vi "BuildRectangularScan_softturn.vi"(0 "VektorCluster":T3={"StartPunkt [m]"={"x"=-3.058577531863264e-05, "y"=1.835670165073038e-05}, "ZeilenIncrement [m]"={"x"=1.0229073667902263e-07, "y"=-4.894247696936301e-07}, "Zeile [m/s]"={"x"=0.21752211986383552, "y"=0.04546254963512117}, "Zeit/Zeile [s]"=0.000225}, 1 "ParameterCluster":T5={"x Pixel"=250, "Lines"=250, "Bidirektional"=TRUE, "AD-Frequency [Hz]"=4000000.0, "Galvo Cycle [s]"=1e-05, "Smartmovedelay [s]"=0.00119, "max.accel. [m/s^2]"=270000.0}) -> (2 "ScanSteuerung":T4(array[cluster])=[{"Zeitpunkt [s]"=0.0, "Wirkung"=enum."Abs", "Kanal"=enum."SMoveTime", "Wert (/s)"=0.0}, {"Zeitpunkt [s]"=0.0, "Wirkung"=enum."Abs", "Kanal"=enum."GalvoX", "Wert (/s)"=-3.058577531863264e-05}, {"Zeitpunkt [s]"=0.0, "Wirkung"=enum."Abs", "Kanal"=enum."GalvoY", "Wert (/s)"=1.835670165073038e-05}, {"Zeitpunkt [s]"=0.0, "Wirkung"=enum."Abs", "Kanal"=enum."Image1X", "Wert (/s)"=0.0}, {"Zeitpunkt [s]"=0.0, "Wirkung"=enum."Abs", "Kanal"=enum."Image1Y", "Wert (/s)"=0.0}, {"Zeitpunkt [s]"=0.0, "Wirkung"=enum."Abs", "Kanal"=enum."Digital", "Wert (/s)"=7.0}, {"Zeitpunkt [s]"=0.0, "Wirkung"=enum."LoopStart", "Kanal"=enum."Loop", "Wert (/s)"=49.0}, {"Zeitpunkt [s]"=0.0, "Wirkung"=enum."Inc", "Kanal"=enum."GalvoX", "Wert (/s)"=0.21752211986383552}, {"Zeitpunkt [s]"=0.0, "Wirkung"=enum."Inc", "Kanal"=enum."GalvoY", "Wert (/s)"=0.04546254963512117}, {"Zeitpunkt [s]"=0.0, "Wirkung"=enum."IncInc", "Kanal"=enum."GalvoX", "Wert (/s)"=0.0}, {"Zeitpunkt [s]"=0.0, "Wirkung"=enum."IncInc", "Kanal"=enum."GalvoY", "Wert (/s)"=0.0}, {"Zeitpunkt [s]"=0.0, "Wirkung"=enum."Inc", "Kanal"=enum."Image1X", "Wert (/s)"=444444.44444444444}, {"Zeitpunkt [s]"=0.00022275, "Wirkung"=enum."Inc", "Kanal"=enum."Image1X", "Wert (/s)"=0.0}, {"Zeitpunkt [s]"=0.000225, "Wirkung"=enum."Inc", "Kanal"=enum."Image1X", "Wert (/s)"=-2315789.47368421}, {"Zeitpunkt [s]"=0.000225, "Wirkung"=enum."Rel", "Kanal"=enum."Image1Y", "Wert (/s)"=1.0}, {"Zeitpunkt [s]"=0.00023, "Wirkung"=enum."Abs", "Kanal"=enum."Digital", "Wert (/s)"=5.0}, {"Zeitpunkt [s]"=0.00023, "Wirkung"=enum."IncInc", "Kanal"=enum."GalvoX", "Wert (/s)"=-146143.4081327828}, {"Zeitpunkt [s]"=0.00023, "Wirkung"=enum."IncInc", "Kanal"=enum."GalvoY", "Wert (/s)"=-32321.565855881716}, {"Zeitpunkt [s]"=0.00025, "Wirkung"=enum."IncInc", "Kanal"=enum."GalvoX", "Wert (/s)"=146143.4081327828}, {"Zeitpunkt [s]"=0.00025, "Wirkung"=enum."IncInc", "Kanal"=enum."GalvoY", "Wert (/s)"=32321.565855881716}, {"Zeitpunkt [s]"=0.00026775000000000003, "Wirkung"=enum."Inc", "Kanal"=enum."Image1X", "Wert (/s)"=0.0}, {"Zeitpunkt [s]"=0.00027, "Wirkung"=enum."Abs", "Kanal"=enum."Digital", "Wert (/s)"=7.0}, {"Zeitpunkt [s]"=0.00027, "Wirkung"=enum."LoopEnd", "Kanal"=enum."Loop", "Wert (/s)"=0.0}, {"Zeitpunkt [s]"=0.01323, "Wirkung"=enum."Inc", "Kanal"=enum."GalvoX", "Wert (/s)"=0.21752211986383552}, {"Zeitpunkt [s]"=0.01323, "Wirkung"=enum."Inc", "Kanal"=enum."GalvoY", "Wert (/s)"=0.04546254963512117}, {"Zeitpunkt [s]"=0.01323, "Wirkung"=enum."IncInc", "Kanal"=enum."GalvoX", "Wert (/s)"=0.0}, {"Zeitpunkt [s]"=0.01323, "Wirkung"=enum."IncInc", "Kanal"=enum."GalvoY", "Wert (/s)"=0.0}, {"Zeitpunkt [s]"=0.01323, "Wirkung"=enum."Inc", "Kanal"=enum."Image1X", "Wert (/s)"=444444.44444444444}, {"Zeitpunkt [s]"=0.013452750000000001, "Wirkung"=enum."Inc", "Kanal"=enum."Image1X", "Wert (/s)"=0.0}, {"Zeitpunkt [s]"=0.013455, "Wirkung"=enum."Inc", "Kanal"=enum."GalvoX", "Wert (/s)"=0.0}, {"Zeitpunkt [s]"=0.013455, "Wirkung"=enum."Inc", "Kanal"=enum."GalvoY", "Wert (/s)"=0.0}, {"Zeitpunkt [s]"=0.013455, "Wirkung"=enum."Abs", "Kanal"=enum."Digital", "Wert (/s)"=0.0}], 3 "Total time":dbl=0.013455, 4 "Line+Turn [s]":dbl=0.00027 format="%^#_6g")   [LabVIEW 2011]
panel:
  out "Galvo tun cycles":dbl=4.0
  out "turn [s] estimate":dbl=0.0004326610977478994
  in  "Neues Zeitraster 2":dbl=1e-05
  in  "Aktiv 2":T1(array[ring])=[enum."GalvoX", enum."GalvoY"]
  out "Fehler":dbl[](array[numeric])=[8.394600298729658e-06, -8.051345387642523e-06]
  out "last value 2":dbl[](array[numeric])=[2.2281337148683577e-05, 4.3766488554712015e-06]
  out "last value":dbl[](array[numeric])=[3.0675937447413235e-05, -3.6746965321713216e-06]
  out "expected classics bidirectioanl":dbl[][](graph)
  in  "Neues Zeitraster":dbl=1e-05
  out "test Graph":dbl[][](graph)=[[-3.058577531863264e-05, 1.835670165073038e-05], [-2.841055411999428e-05, 1.8811327147081594e-05], [-2.6235332921355925e-05, 1.9265952643432807e-05], [-2.4060111722717568e-05, 1.972057813978402e-05], [-2.188489052407921e-05, 2.0175203636135233e-05], [-1.9709669325440853e-05, 2.0629829132486446e-05], [-1.7534448126802496e-05, 2.108445462883766e-05], [-1.535922692816414e-05, 2.153908012518887e-05], [-1.3184005729525784e-05, 2.1993705621540084e-05], [-1.1008784530887429e-05, 2.2448331117891297e-05], [-8.833563332249073e-06, 2.290295661424251e-05], [-6.658342133610718e-06, 2.3357582110593723e-05], [-4.483120934972363e-06, 2.3812207606944936e-05], [-2.3078997363340074e-06, 2.426683310329615e-05], [-1.3267853769565205e-07, 2.472145859964736e-05], [2.0425426609427033e-06, 2.5176084095998575e-05], [4.217763859581059e-06, 2.5630709592349787e-05], [6.392985058219414e-06, 2.6085335088701e-05], [8.56820625685777e-06, 2.6539960585052213e-05], [1.0743427455496125e-05, 2.6994586081403426e-05], [1.291864865413448e-05, 2.744921157775464e-05], [1.5093869852772835e-05, 2.7903837074105852e-05], [1.726909105141119e-05, 2.8358462570457065e-05], [1.9444312250049546e-05, 2.8813088066808278e-05], [2.1619533448687903e-05, 2.926771356315949e-05], [9.180413834047978e-06, 2.649018247392253e-05], [-1.7873046593870224e-05, 2.04804947990974e-05], [-3.0312166208510148e-05, 1.770296370986044e-05], [-2.813694500987179e-05, 1.8157589206211652e-05], [-2.5961723811233434e-05, 1.8612214702562865e-05], [-2.3786502612595077e-05, 1.9066840198914078e-05], [-2.161128141395672e-05, 1.952146569526529e-05], [-1.9436060215318363e-05, 1.9976091191616504e-05], [-1.7260839016680006e-05, 2.0430716687967716e-05], [-1.508561781804165e-05, 2.088534218431893e-05], [-1.2910396619403295e-05, 2.1339967680670142e-05], [-1.073517542076494e-05, 2.1794593177021355e-05], [-8.559954222126584e-06, 2.2249218673372568e-05], [-6.384733023488229e-06, 2.270384416972378e-05], [-4.209511824849874e-06, 2.3158469666074994e-05], [-2.0342906262115183e-06, 2.3613095162426207e-05], [1.40930572426837e-07, 2.406772065877742e-05], [2.3161517710651923e-06, 2.4522346155128633e-05], [4.491372969703548e-06, 2.4976971651479846e-05], [6.666594168341903e-06, 2.543159714783106e-05], [8.841815366980258e-06, 2.588622264418227e-05], [1.1017036565618614e-05, 2.6340848140533484e-05], [1.3192257764256969e-05, 2.6795473636884697e-05], [1.5367478962895323e-05, 2.725009913323591e-05], [1.754270016153368e-05, 2.7704724629587123e-05], [1.9717921360172037e-05, 2.8159350125938336e-05], [2.1893142558810394e-05, 2.861397562228955e-05], [9.454022944170469e-06, 2.5836444533052588e-05], [-1.7599437483747734e-05, 1.9826756858227454e-05], [-3.0038557098387657e-05, 1.7049225768990494e-05], [-2.78633358997493e-05, 1.7503851265341707e-05], [-2.5688114701110943e-05, 1.795847676169292e-05], [-2.3512893502472586e-05, 1.8413102258044132e-05], [-2.133767230383423e-05, 1.8867727754395345e-05], [-1.9162451105195872e-05, 1.9322353250746558e-05], [-1.6987229906557515e-05, 1.977697874709777e-05], [-1.481200870791916e-05, 2.0231604243448984e-05], [-1.2636787509280804e-05, 2.0686229739800197e-05], [-1.0461566310642449e-05, 2.114085523615141e-05], [-8.286345112004094e-06, 2.1595480732502623e-05], [-6.111123913365738e-06, 2.2050106228853836e-05], [-3.935902714727383e-06, 2.250473172520505e-05], [-1.7606815160890276e-06, 2.295935722155626e-05], [4.145396825493277e-07, 2.3413982717907474e-05], [2.589760881187683e-06, 2.3868608214258687e-05], [4.764982079826038e-06, 2.43232337106099e-05], [6.940203278464394e-06, 2.4777859206961113e-05], [9.115424477102749e-06, 2.5232484703312326e-05], [1.1290645675741104e-05, 2.568711019966354e-05], [1.346586687437946e-05, 2.6141735696014752e-05], [1.5641088073017813e-05, 2.6596361192365965e-05], [1.781630927165617e-05, 2.7050986688717178e-05], [1.9991530470294527e-05, 2.750561218506839e-05], [2.2166751668932885e-05, 2.7960237681419603e-05], [9.72763205429296e-06, 2.5182706592182643e-05], [-1.7325828373625243e-05, 1.917301891735751e-05], [-2.9764947988265166e-05, 1.639548782812055e-05], [-2.758972678962681e-05, 1.685011332447176e-05], [-2.5414505590988452e-05, 1.7304738820822974e-05], [-2.3239284392350095e-05, 1.7759364317174187e-05], [-2.106406319371174e-05, 1.82139898135254e-05], [-1.888884199507338e-05, 1.8668615309876613e-05], [-1.6713620796435024e-05, 1.9123240806227826e-05], [-1.4538399597796669e-05, 1.957786630257904e-05], [-1.2363178399158314e-05, 2.003249179893025e-05], [-1.0187957200519958e-05, 2.0487117295281464e-05], [-8.012736001881603e-06, 2.0941742791632677e-05], [-5.8375148032432476e-06, 2.139636828798389e-05], [-3.6622936046048922e-06, 2.1850993784335103e-05], [-1.4870724059665369e-06, 2.2305619280686316e-05], [6.881487926718185e-07, 2.276024477703753e-05], [2.863369991310174e-06, 2.3214870273388742e-05], [5.038591189948529e-06, 2.3669495769739955e-05], [7.2138123885868845e-06, 2.4124121266091168e-05], [9.38903358722524e-06, 2.457874676244238e-05], [1.1564254785863595e-05, 2.5033372258793593e-05], [1.373947598450195e-05, 2.5487997755144806e-05], [1.5914697183140304e-05, 2.594262325149602e-05], [1.808991838177866e-05, 2.6397248747847232e-05], [2.0265139580417018e-05, 2.6851874244198445e-05], [2.2440360779055375e-05, 2.7306499740549658e-05], [1.000124116441545e-05, 2.4528968651312697e-05], [-1.7052219263502752e-05, 1.8519280976487563e-05], [-2.9491338878142676e-05, 1.5741749887250603e-05], [-2.731611767950432e-05, 1.6196375383601816e-05], [-2.514089648086596e-05, 1.665100087995303e-05], [-2.2965675282227605e-05, 1.710562637630424e-05], [-2.0790454083589248e-05, 1.7560251872655455e-05], [-1.861523288495089e-05, 1.8014877369006667e-05], [-1.6440011686312534e-05, 1.846950286535788e-05], [-1.4264790487674178e-05, 1.8924128361709093e-05], [-1.2089569289035823e-05, 1.9378753858060306e-05], [-9.914348090397468e-06, 1.983337935441152e-05], [-7.739126891759112e-06, 2.0288004850762732e-05], [-5.563905693120757e-06, 2.0742630347113945e-05], [-3.3886844944824015e-06, 2.1197255843465158e-05], [-1.2134632958440462e-06, 2.165188133981637e-05], [9.617579027943092e-07, 2.2106506836167584e-05], [3.1369791014326645e-06, 2.2561132332518797e-05], [5.31220030007102e-06, 2.301575782887001e-05], [7.487421498709375e-06, 2.3470383325221222e-05], [9.66264269734773e-06, 2.3925008821572435e-05], [1.1837863895986086e-05, 2.4379634317923648e-05], [1.4013085094624441e-05, 2.483425981427486e-05], [1.6188306293262795e-05, 2.5288885310626074e-05], [1.8363527491901152e-05, 2.5743510806977287e-05], [2.053874869053951e-05, 2.61981363033285e-05], [2.2713969889177866e-05, 2.6652761799679713e-05], [1.027485027453794e-05, 2.3875230710442752e-05], [-1.677861015338026e-05, 1.7865543035617618e-05], [-2.9217729768020185e-05, 1.5088011946380658e-05], [-2.7042508569381828e-05, 1.554263744273187e-05], [-2.486728737074347e-05, 1.5997262939083083e-05], [-2.2692066172105114e-05, 1.6451888435434296e-05], [-2.0516844973466757e-05, 1.690651393178551e-05], [-1.83416237748284e-05, 1.7361139428136722e-05], [-1.6166402576190043e-05, 1.7815764924487935e-05], [-1.3991181377551687e-05, 1.8270390420839148e-05], [-1.1815960178913332e-05, 1.872501591719036e-05], [-9.640738980274977e-06, 1.9179641413541574e-05], [-7.4655177816366214e-06, 1.9634266909892787e-05], [-5.290296582998266e-06, 2.0088892406244e-05], [-3.1150753843599108e-06, 2.0543517902595212e-05], [-9.398541857215554e-07, 2.0998143398946425e-05], [1.2353670129168e-06, 2.1452768895297638e-05], [3.4105882115551553e-06, 2.190739439164885e-05], [5.585809410193511e-06, 2.2362019888000064e-05], [7.761030608831866e-06, 2.2816645384351277e-05], [9.936251807470221e-06, 2.327127088070249e-05], [1.2111473006108577e-05, 2.3725896377053703e-05], [1.4286694204746932e-05, 2.4180521873404916e-05], [1.6461915403385286e-05, 2.463514736975613e-05], [1.8637136602023643e-05, 2.508977286610734e-05], [2.0812357800662e-05, 2.5544398362458554e-05], [2.2987578999300357e-05, 2.5999023858809767e-05], [1.0548459384660432e-05, 2.3221492769572807e-05], [-1.650500104325777e-05, 1.7211805094747673e-05], [-2.8944120657897694e-05, 1.4434274005510712e-05], [-2.6768899459259337e-05, 1.4888899501861923e-05], [-2.459367826062098e-05, 1.5343524998213135e-05], [-2.2418457061982623e-05, 1.5798150494564348e-05], [-2.0243235863344266e-05, 1.625277599091556e-05], [-1.806801466470591e-05, 1.6707401487266773e-05], [-1.5892793466067552e-05, 1.7162026983617986e-05], [-1.3717572267429197e-05, 1.76166524799692e-05], [-1.1542351068790841e-05, 1.8071277976320412e-05], [-9.367129870152486e-06, 1.8525903472671625e-05], [-7.191908671514131e-06, 1.8980528969022838e-05], [-5.016687472875775e-06, 1.943515446537405e-05], [-2.84146627423742e-06, 1.9889779961725264e-05], [-6.662450755990647e-07, 2.0344405458076477e-05], [1.5089761230392907e-06, 2.079903095442769e-05], [3.684197321677646e-06, 2.1253656450778902e-05], [5.859418520316001e-06, 2.1708281947130115e-05], [8.034639718954357e-06, 2.2162907443481328e-05], [1.0209860917592712e-05, 2.261753293983254e-05], [1.2385082116231067e-05, 2.3072158436183754e-05], [1.4560303314869423e-05, 2.3526783932534967e-05], [1.6735524513507776e-05, 2.398140942888618e-05], [1.8910745712146133e-05, 2.4436034925237393e-05], [2.108596691078449e-05, 2.4890660421588606e-05], [2.3261188109422847e-05, 2.534528591793982e-05], [1.0822068494782922e-05, 2.2567754828702858e-05], [-1.623139193313528e-05, 1.6558067153877727e-05], [-2.8670511547775204e-05, 1.3780536064640767e-05], [-2.6495290349136847e-05, 1.4235161560991978e-05], [-2.432006915049849e-05, 1.468978705734319e-05], [-2.2144847951860132e-05, 1.51444125536944e-05], [-1.9969626753221775e-05, 1.559903805004561e-05], [-1.779440555458342e-05, 1.6053663546396825e-05], [-1.561918435594506e-05, 1.6508289042748037e-05], [-1.3443963157306706e-05, 1.696291453909925e-05], [-1.126874195866835e-05, 1.7417540035450463e-05], [-9.093520760029995e-06, 1.7872165531801676e-05], [-6.91829956139164e-06, 1.832679102815289e-05], [-4.743078362753285e-06, 1.8781416524504102e-05], [-2.5678571641149293e-06, 1.9236042020855315e-05], [-3.9263596547657396e-07, 1.9690667517206528e-05], [1.7825852331617814e-06, 2.014529301355774e-05], [3.957806431800137e-06, 2.0599918509908954e-05], [6.133027630438492e-06, 2.1054544006260167e-05], [8.308248829076847e-06, 2.150916950261138e-05], [1.0483470027715203e-05, 2.1963794998962592e-05], [1.2658691226353558e-05, 2.2418420495313805e-05], [1.4833912424991913e-05, 2.2873045991665018e-05], [1.7009133623630267e-05, 2.332767148801623e-05], [1.9184354822268624e-05, 2.3782296984367444e-05], [2.135957602090698e-05, 2.4236922480718657e-05], [2.3534797219545338e-05, 2.469154797706987e-05], [1.1095677604905413e-05, 2.191401688783291e-05], [-1.595778282301279e-05, 1.5904329213007775e-05], [-2.8396902437652713e-05, 1.3126798123770815e-05], [-2.6221681239014356e-05, 1.3581423620122026e-05], [-2.4046460040376e-05, 1.4036049116473237e-05], [-2.1871238841737642e-05, 1.4490674612824448e-05], [-1.9696017643099285e-05, 1.494530010917566e-05], [-1.7520796444460928e-05, 1.5399925605526872e-05], [-1.534557524582257e-05, 1.5854551101878085e-05], [-1.3170354047184215e-05, 1.6309176598229298e-05], [-1.099513284854586e-05, 1.676380209458051e-05], [-8.819911649907505e-06, 1.7218427590931724e-05], [-6.644690451269149e-06, 1.7673053087282937e-05], [-4.469469252630794e-06, 1.812767858363415e-05], [-2.2942480539924386e-06, 1.8582304079985363e-05], [-1.1902685535408323e-07, 1.9036929576336576e-05], [2.056194343284272e-06, 1.949155507268779e-05], [4.2314155419226275e-06, 1.9946180569039e-05], [6.406636740560983e-06, 2.0400806065390214e-05], [8.581857939199338e-06, 2.0855431561741427e-05], [1.0757079137837693e-05, 2.131005705809264e-05], [1.2932300336476049e-05, 2.1764682554443853e-05], [1.5107521535114404e-05, 2.2219308050795066e-05], [1.7282742733752758e-05, 2.267393354714628e-05], [1.9457963932391115e-05, 2.3128559043497492e-05], [2.1633185131029472e-05, 2.3583184539848705e-05], [2.380840632966783e-05, 2.4037810036199918e-05], [1.1369286715027904e-05, 2.1260278946962957e-05], [-1.56841737128903e-05, 1.5250591272137825e-05], [-2.8123293327530222e-05, 1.2473060182900864e-05], [-2.5948072128891865e-05, 1.2927685679252075e-05], [-2.3772850930253508e-05, 1.3382311175603287e-05], [-2.159762973161515e-05, 1.3836936671954498e-05], [-1.9422408532976794e-05, 1.4291562168305709e-05], [-1.7247187334338437e-05, 1.474618766465692e-05], [-1.5071966135700082e-05, 1.5200813161008132e-05], [-1.2896744937061726e-05, 1.5655438657359343e-05], [-1.0721523738423371e-05, 1.6110064153710556e-05], [-8.546302539785016e-06, 1.656468965006177e-05], [-6.37108134114666e-06, 1.701931514641298e-05], [-4.195860142508305e-06, 1.7473940642764194e-05], [-2.0206389438699495e-06, 1.7928566139115407e-05], [1.545822547684058e-07, 1.838319163546662e-05], [2.329803453406761e-06, 1.8837817131817833e-05], [4.5050246520451165e-06, 1.9292442628169046e-05], [6.680245850683472e-06, 1.974706812452026e-05], [8.855467049321827e-06, 2.0201693620871472e-05], [1.1030688247960183e-05, 2.0656319117222685e-05], [1.3205909446598538e-05, 2.1110944613573898e-05], [1.538113064523689e-05, 2.156557010992511e-05], [1.755635184387525e-05, 2.2020195606276323e-05], [1.9731573042513606e-05, 2.2474821102627536e-05], [2.1906794241151963e-05, 2.292944659897875e-05], [2.408201543979032e-05, 2.3384072095329962e-05], [1.1642895825150394e-05, 2.0606541006093e-05], [-1.5410564602767808e-05, 1.459685333126787e-05], [-2.784968421740773e-05, 1.1819322242030909e-05], [-2.5674463018769374e-05, 1.227394773838212e-05], [-2.3499241820131017e-05, 1.2728573234733331e-05], [-2.132402062149266e-05, 1.3183198731084542e-05], [-1.9148799422854303e-05, 1.3637824227435754e-05], [-1.6973578224215946e-05, 1.4092449723786965e-05], [-1.479835702557759e-05, 1.4547075220138176e-05], [-1.2623135826939235e-05, 1.5001700716489387e-05], [-1.044791462830088e-05, 1.54563262128406e-05], [-8.272693429662525e-06, 1.5910951709191813e-05], [-6.0974722310241695e-06, 1.6365577205543026e-05], [-3.922251032385814e-06, 1.682020270189424e-05], [-1.7470298337474588e-06, 1.7274828198245452e-05], [4.2819136489089654e-07, 1.7729453694596665e-05], [2.603412563529252e-06, 1.8184079190947878e-05], [4.778633762167607e-06, 1.863870468729909e-05], [6.9538549608059626e-06, 1.9093330183650303e-05], [9.129076159444318e-06, 1.9547955680001516e-05], [1.1304297358082673e-05, 2.000258117635273e-05], [1.3479518556721029e-05, 2.0457206672703942e-05], [1.5654739755359382e-05, 2.0911832169055155e-05], [1.782996095399774e-05, 2.1366457665406368e-05], [2.0005182152636096e-05, 2.182108316175758e-05], [2.2180403351274453e-05, 2.2275708658108794e-05], [2.435562454991281e-05, 2.2730334154460007e-05], [1.1916504935272885e-05, 1.9952803065223046e-05], [-1.5136955492645319e-05, 1.3943115390397914e-05], [-2.757607510728524e-05, 1.1165584301160953e-05], [-2.5400853908646884e-05, 1.1620209797512164e-05], [-2.3225632710008527e-05, 1.2074835293863376e-05], [-2.105041151137017e-05, 1.2529460790214587e-05], [-1.8875190312731812e-05, 1.2984086286565798e-05], [-1.6699969114093455e-05, 1.343871178291701e-05], [-1.45247479154551e-05, 1.389333727926822e-05], [-1.2349526716816745e-05, 1.4347962775619432e-05], [-1.017430551817839e-05, 1.4802588271970643e-05], [-7.999084319540034e-06, 1.5257213768321854e-05], [-5.823863120901679e-06, 1.5711839264673067e-05], [-3.6486419222633234e-06, 1.616646476102428e-05], [-1.473420723624968e-06, 1.6621090257375493e-05], [7.018004750133873e-07, 1.7075715753726706e-05], [2.8770216736517426e-06, 1.753034125007792e-05], [5.052242872290098e-06, 1.798496674642913e-05], [7.227464070928453e-06, 1.8439592242780344e-05], [9.402685269566809e-06, 1.8894217739131557e-05], [1.1577906468205164e-05, 1.934884323548277e-05], [1.375312766684352e-05, 1.9803468731833983e-05], [1.5928348865481873e-05, 2.0258094228185196e-05], [1.810357006412023e-05, 2.071271972453641e-05], [2.0278791262758587e-05, 2.1167345220887622e-05], [2.2454012461396944e-05, 2.1621970717238835e-05], [2.46292336600353e-05, 2.2076596213590048e-05], [1.2190114045395376e-05, 1.9299065124353087e-05], [-1.4863346382522828e-05, 1.3289377449527955e-05], [-2.730246599716275e-05, 1.0511846360290994e-05], [-2.5127244798524393e-05, 1.0966471856642205e-05], [-2.2952023599886036e-05, 1.1421097352993417e-05], [-2.077680240124768e-05, 1.1875722849344628e-05], [-1.8601581202609322e-05, 1.2330348345695839e-05], [-1.6426360003970965e-05, 1.278497384204705e-05], [-1.425113880533261e-05, 1.3239599338398262e-05], [-1.2075917606694254e-05, 1.3694224834749473e-05], [-9.900696408055899e-06, 1.4148850331100684e-05], [-7.725475209417543e-06, 1.4603475827451895e-05], [-5.550254010779188e-06, 1.5058101323803106e-05], [-3.3750328121408327e-06, 1.5512726820154318e-05], [-1.1998116135024773e-06, 1.596735231650553e-05], [9.75409585135878e-07, 1.6421977812856743e-05], [3.1506307837742333e-06, 1.6876603309207956e-05], [5.325851982412589e-06, 1.733122880555917e-05], [7.501073181050944e-06, 1.7785854301910382e-05], [9.6762943796893e-06, 1.8240479798261595e-05], [1.1851515578327655e-05, 1.8695105294612808e-05], [1.402673677696601e-05, 1.914973079096402e-05], [1.6201957975604364e-05, 1.9604356287315234e-05], [1.837717917424272e-05, 2.0058981783666447e-05], [2.0552400372881078e-05, 2.051360728001766e-05], [2.2727621571519435e-05, 2.0968232776368872e-05], [2.4902842770157792e-05, 2.1422858272720085e-05], [1.2463723155517867e-05, 1.8645327183483125e-05], [-1.4589737272400337e-05, 1.2635639508657992e-05], [-2.702885688704026e-05, 9.858108419421032e-06], [-2.4853635688401902e-05, 1.0312733915772243e-05], [-2.2678414489763545e-05, 1.0767359412123454e-05], [-2.0503193291125188e-05, 1.1221984908474666e-05], [-1.832797209248683e-05, 1.1676610404825877e-05], [-1.6152750893848474e-05, 1.2131235901177088e-05], [-1.3977529695210119e-05, 1.25858613975283e-05], [-1.1802308496571763e-05, 1.304048689387951e-05], [-9.627087297933408e-06, 1.3495112390230722e-05], [-7.451866099295053e-06, 1.3949737886581933e-05], [-5.276644900656697e-06, 1.4404363382933144e-05], [-3.101423702018342e-06, 1.4858988879284355e-05], [-9.262025033799866e-07, 1.5313614375635568e-05], [1.2490186952583687e-06, 1.576823987198678e-05], [3.424239893896724e-06, 1.6222865368337994e-05], [5.599461092535079e-06, 1.6677490864689207e-05], [7.774682291173435e-06, 1.713211636104042e-05], [9.94990348981179e-06, 1.7586741857391633e-05], [1.2125124688450145e-05, 1.8041367353742846e-05], [1.43003458870885e-05, 1.849599285009406e-05], [1.6475567085726854e-05, 1.895061834644527e-05], [1.865078828436521e-05, 1.9405243842796484e-05], [2.082600948300357e-05, 1.9859869339147697e-05], [2.3001230681641926e-05, 2.031449483549891e-05], [2.5176451880280283e-05, 2.0769120331850123e-05], [1.2737332265640357e-05, 1.7991589242613162e-05], [-1.4316128162277847e-05, 1.198190156778803e-05], [-2.675524777691777e-05, 9.20437047855107e-06], [-2.458002657827941e-05, 9.658995974902281e-06], [-2.2404805379641054e-05, 1.0113621471253492e-05], [-2.0229584181002697e-05, 1.0568246967604703e-05], [-1.805436298236434e-05, 1.1022872463955914e-05], [-1.5879141783725983e-05, 1.1477497960307126e-05], [-1.3703920585087628e-05, 1.1932123456658337e-05], [-1.1528699386449273e-05, 1.2386748953009548e-05], [-9.353478187810917e-06, 1.284137444936076e-05], [-7.178256989172562e-06, 1.329599994571197e-05], [-5.0030357905342065e-06, 1.3750625442063182e-05], [-2.827814591895851e-06, 1.4205250938414393e-05], [-6.525933932574959e-07, 1.4659876434765604e-05], [1.5226278053808595e-06, 1.5114501931116815e-05], [3.697849004019215e-06, 1.5569127427468028e-05], [5.87307020265757e-06, 1.602375292381924e-05], [8.048291401295925e-06, 1.6478378420170454e-05], [1.022351259993428e-05, 1.6933003916521667e-05], [1.2398733798572636e-05, 1.738762941287288e-05], [1.4573954997210992e-05, 1.7842254909224093e-05], [1.6749176195849345e-05, 1.8296880405575306e-05], [1.8924397394487702e-05, 1.875150590192652e-05], [2.109961859312606e-05, 1.920613139827773e-05], [2.3274839791764416e-05, 1.9660756894628944e-05], [2.5450060990402773e-05, 2.0115382390980157e-05], [1.3010941375762848e-05, 1.7337851301743197e-05], [-1.4042519052155356e-05, 1.1328163626918064e-05], [-2.6481638666795278e-05, 8.550632537681104e-06], [-2.430641746815692e-05, 9.005258034032315e-06], [-2.2131196269518564e-05, 9.459883530383526e-06], [-1.9955975070880207e-05, 9.914509026734738e-06], [-1.778075387224185e-05, 1.0369134523085949e-05], [-1.5605532673603493e-05, 1.082376001943716e-05], [-1.3430311474965137e-05, 1.1278385515788371e-05], [-1.1255090276326782e-05, 1.1733011012139582e-05], [-9.079869077688426e-06, 1.2187636508490794e-05], [-6.904647879050071e-06, 1.2642262004842005e-05], [-4.729426680411716e-06, 1.3096887501193216e-05], [-2.5542054817733605e-06, 1.3551512997544427e-05], [-3.7898428313500514e-07, 1.4006138493895638e-05], [1.7962369155033502e-06, 1.446076399024685e-05], [3.9714581141417055e-06, 1.4915389486598061e-05], [6.146679312780061e-06, 1.5370014982949272e-05], [8.321900511418416e-06, 1.5824640479300485e-05], [1.0497121710056772e-05, 1.6279265975651698e-05], [1.2672342908695127e-05, 1.673389147200291e-05], [1.4847564107333482e-05, 1.7188516968354124e-05], [1.7022785305971836e-05, 1.7643142464705337e-05], [1.9198006504610193e-05, 1.809776796105655e-05], [2.137322770324855e-05, 1.8552393457407762e-05], [2.3548448901886907e-05, 1.9007018953758975e-05], [2.5723670100525264e-05, 1.9461644450110188e-05], [1.3284550485885339e-05, 1.6684113360873228e-05], [-1.3768909942032865e-05, 1.0674425686048095e-05], [-2.6208029556672787e-05, 7.896894596811135e-06], [-2.403280835803443e-05, 8.351520093162346e-06], [-2.1857587159396073e-05, 8.806145589513557e-06], [-1.9682365960757716e-05, 9.260771085864769e-06], [-1.750714476211936e-05, 9.71539658221598e-06], [-1.5331923563481002e-05, 1.0170022078567191e-05], [-1.3156702364842646e-05, 1.0624647574918402e-05], [-1.0981481166204291e-05, 1.1079273071269613e-05], [-8.806259967565936e-06, 1.1533898567620825e-05], [-6.63103876892758e-06, 1.1988524063972036e-05], [-4.455817570289225e-06, 1.2443149560323247e-05], [-2.2805963716508697e-06, 1.2897775056674458e-05], [-1.053751730125144e-07, 1.335240055302567e-05], [2.069846025625841e-06, 1.380702604937688e-05], [4.245067224264196e-06, 1.4261651545728092e-05], [6.420288422902552e-06, 1.4716277042079303e-05], [8.595509621540907e-06, 1.5170902538430514e-05], [1.0770730820179262e-05, 1.5625528034781725e-05], [1.2945952018817618e-05, 1.608015353113294e-05], [1.5121173217455973e-05, 1.653477902748415e-05], [1.7296394416094327e-05, 1.6989404523835364e-05], [1.9471615614732684e-05, 1.7444030020186577e-05], [2.164683681337104e-05, 1.789865551653779e-05], [2.3822058012009398e-05, 1.8353281012889003e-05], [2.5997279210647755e-05, 1.8807906509240216e-05], [1.355815959600783e-05, 1.6030375420003255e-05], [-1.3495300831910374e-05, 1.0020687745178123e-05], [-2.5934420446550296e-05, 7.243156655941162e-06], [-2.375919924791194e-05, 7.697782152292374e-06], [-2.1583978049273582e-05, 8.152407648643585e-06], [-1.9408756850635225e-05, 8.607033144994796e-06], [-1.7233535651996868e-05, 9.061658641346007e-06], [-1.5058314453358513e-05, 9.516284137697218e-06], [-1.2883093254720157e-05, 9.97090963404843e-06], [-1.0707872056081802e-05, 1.0425535130399641e-05], [-8.532650857443447e-06, 1.0880160626750852e-05], [-6.357429658805091e-06, 1.1334786123102063e-05], [-4.182208460166736e-06, 1.1789411619453274e-05], [-2.0069872615283807e-06, 1.2244037115804486e-05], [1.6823393710997463e-07, 1.2698662612155697e-05], [2.34345513574833e-06, 1.3153288108506908e-05], [4.518676334386685e-06, 1.360791360485812e-05], [6.693897533025041e-06, 1.406253910120933e-05], [8.869118731663396e-06, 1.4517164597560542e-05], [1.1044339930301751e-05, 1.4971790093911753e-05], [1.3219561128940107e-05, 1.5426415590262966e-05], [1.539478232757846e-05, 1.588104108661418e-05], [1.7570003526216817e-05, 1.633566658296539e-05], [1.9745224724855174e-05, 1.6790292079316605e-05], [2.192044592349353e-05, 1.7244917575667817e-05], [2.409566712213189e-05, 1.769954307201903e-05], [2.6270888320770245e-05, 1.8154168568370243e-05], [1.383176870613032e-05, 1.5376637479133283e-05], [-1.3221691721787884e-05, 9.36694980430815e-06], [-2.5660811336427805e-05, 6.58941871507119e-06], [-2.348559013778945e-05, 7.044044211422402e-06], [-2.131036893915109e-05, 7.498669707773614e-06], [-1.9135147740512734e-05, 7.953295204124825e-06], [-1.6959926541874377e-05, 8.407920700476036e-06], [-1.4784705343236022e-05, 8.862546196827248e-06], [-1.2609484144597667e-05, 9.317171693178459e-06], [-1.0434262945959311e-05, 9.77179718952967e-06], [-8.259041747320956e-06, 1.0226422685880881e-05], [-6.083820548682601e-06, 1.0681048182232093e-05], [-3.908599350044245e-06, 1.1135673678583304e-05], [-1.73337815140589e-06, 1.1590299174934515e-05], [4.4184304723246537e-07, 1.2044924671285726e-05], [2.6170642458708207e-06, 1.2499550167636937e-05], [4.792285444509176e-06, 1.2954175663988149e-05], [6.967506643147531e-06, 1.340880116033936e-05], [9.142727841785887e-06, 1.3863426656690571e-05], [1.1317949040424242e-05, 1.4318052153041782e-05], [1.3493170239062597e-05, 1.4772677649392993e-05], [1.566839143770095e-05, 1.5227303145744205e-05], [1.7843612636339308e-05, 1.5681928642095416e-05], [2.0018833834977665e-05, 1.613655413844663e-05], [2.2194055033616022e-05, 1.659117963479784e-05], [2.436927623225438e-05, 1.7045805131149055e-05], [2.6544497430892736e-05, 1.7500430627500267e-05], [1.4105377816252811e-05, 1.4722899538263307e-05], [-1.2948082611665393e-05, 8.713211863438175e-06], [-2.5387202226305315e-05, 5.935680774201214e-06], [-2.3211981027666958e-05, 6.390306270552426e-06], [-2.10367598290286e-05, 6.844931766903638e-06], [-1.8861538630390244e-05, 7.29955726325485e-06], [-1.6686317431751887e-05, 7.754182759606062e-06], [-1.4511096233113531e-05, 8.208808255957273e-06], [-1.2335875034475176e-05, 8.663433752308485e-06], [-1.016065383583682e-05, 9.118059248659696e-06], [-7.985432637198465e-06, 9.572684745010907e-06], [-5.81021143856011e-06, 1.0027310241362118e-05], [-3.6349902399217546e-06, 1.048193573771333e-05], [-1.4597690412833992e-06, 1.093656123406454e-05], [7.154521573549561e-07, 1.1391186730415752e-05], [2.8906733559933114e-06, 1.1845812226766963e-05], [5.065894554631667e-06, 1.2300437723118174e-05], [7.241115753270022e-06, 1.2755063219469386e-05], [9.416336951908377e-06, 1.3209688715820597e-05], [1.1591558150546733e-05, 1.3664314212171808e-05], [1.3766779349185088e-05, 1.411893970852302e-05], [1.5942000547823442e-05, 1.457356520487423e-05], [1.81172217464618e-05, 1.5028190701225442e-05], [2.0292442945100156e-05, 1.5482816197576653e-05], [2.2467664143738513e-05, 1.5937441693927866e-05], [2.464288534237687e-05, 1.639206719027908e-05], [2.6818106541015227e-05, 1.684669268663029e-05], [1.4378986926375302e-05, 1.4069161597393331e-05], [-1.2674473501542902e-05, 8.059473922568199e-06], [-2.5113593116182824e-05, 5.281942833331238e-06], [-2.2938371917544467e-05, 5.73656832968245e-06], [-2.076315071890611e-05, 6.191193826033662e-06], [-1.8587929520267753e-05, 6.645819322384874e-06], [-1.6412708321629396e-05, 7.1004448187360864e-06], [-1.423748712299104e-05, 7.5550703150872985e-06], [-1.2062265924352685e-05, 8.00969581143851e-06], [-9.88704472571433e-06, 8.464321307789722e-06], [-7.711823527075975e-06, 8.918946804140933e-06], [-5.536602328437619e-06, 9.373572300492144e-06], [-3.361381129799264e-06, 9.828197796843355e-06], [-1.1861599311609085e-06, 1.0282823293194567e-05], [9.890612674774468e-07, 1.0737448789545778e-05], [3.164282466115802e-06, 1.1192074285896989e-05], [5.3395036647541575e-06, 1.16466997822482e-05], [7.514724863392513e-06, 1.2101325278599411e-05], [9.689946062030868e-06, 1.2555950774950623e-05], [1.1865167260669224e-05, 1.3010576271301834e-05], [1.4040388459307579e-05, 1.3465201767653045e-05], [1.6215609657945933e-05, 1.3919827264004256e-05], [1.839083085658429e-05, 1.4374452760355467e-05], [2.0566052055222647e-05, 1.4829078256706679e-05], [2.2741273253861004e-05, 1.528370375305789e-05], [2.491649445249936e-05, 1.5738329249409103e-05], [2.7091715651137718e-05, 1.6192954745760316e-05], [1.4652596036497793e-05, 1.3415423656523355e-05], [-1.2400864391420411e-05, 7.405735981698223e-06], [-2.4839984006060333e-05, 4.628204892461262e-06], [-2.2664762807421976e-05, 5.082830388812474e-06], [-2.048954160878362e-05, 5.5374558851636865e-06], [-1.8314320410145262e-05, 5.9920813815148985e-06], [-1.6139099211506905e-05, 6.4467068778661106e-06], [-1.396387801286855e-05, 6.901332374217323e-06], [-1.1788656814230194e-05, 7.355957870568535e-06], [-9.613435615591839e-06, 7.810583366919746e-06], [-7.438214416953484e-06, 8.265208863270957e-06], [-5.2629932183151285e-06, 8.719834359622168e-06], [-3.087772019676773e-06, 9.17445985597338e-06], [-9.125508210384178e-07, 9.62908535232459e-06], [1.2626703775999376e-06, 1.0083710848675802e-05], [3.437891576238293e-06, 1.0538336345027013e-05], [5.613112774876648e-06, 1.0992961841378224e-05], [7.788333973515004e-06, 1.1447587337729436e-05], [9.963555172153359e-06, 1.1902212834080647e-05], [1.2138776370791714e-05, 1.2356838330431858e-05], [1.431399756943007e-05, 1.281146382678307e-05], [1.6489218768068423e-05, 1.326608932313428e-05], [1.866443996670678e-05, 1.3720714819485492e-05], [2.0839661165345137e-05, 1.4175340315836703e-05], [2.3014882363983494e-05, 1.4629965812187914e-05], [2.519010356262185e-05, 1.5084591308539125e-05], [2.736532476126021e-05, 1.5539216804890336e-05], [1.4926205146620283e-05, 1.2761685715653376e-05], [-1.212725528129792e-05, 6.751998040828244e-06], [-2.4566374895937843e-05, 3.974466951591283e-06], [-2.2391153697299486e-05, 4.429092447942495e-06], [-2.021593249866113e-05, 4.883717944293707e-06], [-1.804071130002277e-05, 5.338343440644919e-06], [-1.5865490101384414e-05, 5.792968936996131e-06], [-1.3690268902746059e-05, 6.247594433347343e-06], [-1.1515047704107704e-05, 6.7022199296985554e-06], [-9.339826505469348e-06, 7.1568454260497675e-06], [-7.164605306830993e-06, 7.6114709224009795e-06], [-4.989384108192638e-06, 8.06609641875219e-06], [-2.8141629095542824e-06, 8.520721915103402e-06], [-6.38941710915927e-07, 8.975347411454613e-06], [1.5362794877224283e-06, 9.429972907805824e-06], [3.7115006863607836e-06, 9.884598404157036e-06], [5.886721884999139e-06, 1.0339223900508247e-05], [8.061943083637494e-06, 1.0793849396859458e-05], [1.023716428227585e-05, 1.124847489321067e-05], [1.2412385480914205e-05, 1.170310038956188e-05], [1.458760667955256e-05, 1.2157725885913092e-05], [1.6762827878190914e-05, 1.2612351382264303e-05], [1.893804907682927e-05, 1.3066976878615514e-05], [2.1113270275467628e-05, 1.3521602374966725e-05], [2.3288491474105985e-05, 1.3976227871317936e-05], [2.5463712672744342e-05, 1.4430853367669148e-05], [2.76389338713827e-05, 1.4885478864020359e-05], [1.5199814256742774e-05, 1.2107947774783398e-05], [-1.185364617117543e-05, 6.098260099958266e-06], [-2.4292765785815352e-05, 3.320729010721306e-06], [-2.2117544587176995e-05, 3.7753545070725176e-06], [-1.9942323388538638e-05, 4.22998000342373e-06], [-1.776710218990028e-05, 4.684605499774942e-06], [-1.5591880991261924e-05, 5.139230996126154e-06], [-1.3416659792623568e-05, 5.593856492477366e-06], [-1.1241438593985213e-05, 6.048481988828578e-06], [-9.066217395346858e-06, 6.50310748517979e-06], [-6.890996196708502e-06, 6.957732981531002e-06], [-4.715774998070147e-06, 7.412358477882214e-06], [-2.5405537994317917e-06, 7.866983974233426e-06], [-3.653326007934363e-07, 8.321609470584637e-06], [1.809888597844919e-06, 8.776234966935849e-06], [3.985109796483274e-06, 9.23086046328706e-06], [6.16033099512163e-06, 9.685485959638271e-06], [8.335552193759985e-06, 1.0140111455989482e-05], [1.051077339239834e-05, 1.0594736952340693e-05], [1.2685994591036696e-05, 1.1049362448691905e-05], [1.4861215789675051e-05, 1.1503987945043116e-05], [1.7036436988313405e-05, 1.1958613441394327e-05], [1.9211658186951762e-05, 1.2413238937745538e-05], [2.138687938559012e-05, 1.286786443409675e-05], [2.3562100584228476e-05, 1.332248993044796e-05], [2.5737321782866833e-05, 1.3777115426799172e-05], [2.791254298150519e-05, 1.4231740923150383e-05], [1.5473423366865266e-05, 1.1454209833913422e-05], [-1.1580037061052938e-05, 5.44452215908829e-06], [-2.401915667569286e-05, 2.66699106985133e-06], [-2.1843935477054504e-05, 3.1216165662025417e-06], [-1.9668714278416147e-05, 3.5762420625537534e-06], [-1.749349307977779e-05, 4.030867558904965e-06], [-1.5318271881139433e-05, 4.485493055256177e-06], [-1.3143050682501078e-05, 4.940118551607389e-06], [-1.0967829483862722e-05, 5.394744047958601e-06], [-8.792608285224367e-06, 5.849369544309813e-06], [-6.617387086586012e-06, 6.303995040661025e-06], [-4.442165887947656e-06, 6.758620537012237e-06], [-2.266944689309301e-06, 7.213246033363449e-06], [-9.172349067094558e-08, 7.667871529714661e-06], [2.0834977079674098e-06, 8.122497026065873e-06], [4.258718906605765e-06, 8.577122522417084e-06], [6.4339401052441204e-06, 9.031748018768295e-06], [8.609161303882476e-06, 9.486373515119506e-06], [1.0784382502520831e-05, 9.940999011470717e-06], [1.2959603701159186e-05, 1.0395624507821929e-05], [1.5134824899797542e-05, 1.085025000417314e-05], [1.7310046098435895e-05, 1.1304875500524351e-05], [1.9485267297074252e-05, 1.1759500996875562e-05], [2.166048849571261e-05, 1.2214126493226774e-05], [2.3835709694350967e-05, 1.2668751989577985e-05], [2.6010930892989324e-05, 1.3123377485929196e-05], [2.818615209162768e-05, 1.3578002982280407e-05], [1.5747032476987757e-05, 1.0800471893043447e-05], [-1.1306427950930447e-05, 4.790784218218314e-06], [-2.374554756557037e-05, 2.0132531289813542e-06], [-2.1570326366932013e-05, 2.467878625332566e-06], [-1.9395105168293656e-05, 2.9225041216837775e-06], [-1.72198839696553e-05, 3.377129618034989e-06], [-1.5044662771016944e-05, 3.831755114386201e-06], [-1.2869441572378589e-05, 4.286380610737413e-06], [-1.0694220373740233e-05, 4.741006107088625e-06], [-8.518999175101878e-06, 5.195631603439837e-06], [-6.3437779764635226e-06, 5.650257099791049e-06], [-4.168556777825167e-06, 6.1048825961422615e-06], [-1.993335579186812e-06, 6.5595080924934735e-06], [1.8188561945154346e-07, 7.014133588844686e-06], [2.357106818089899e-06, 7.468759085195898e-06], [4.532328016728254e-06, 7.92338458154711e-06], [6.7075492153666095e-06, 8.378010077898321e-06], [8.882770414004965e-06, 8.832635574249532e-06], [1.105799161264332e-05, 9.287261070600743e-06], [1.3233212811281675e-05, 9.741886566951955e-06], [1.540843400992003e-05, 1.0196512063303166e-05], [1.7583655208558386e-05, 1.0651137559654377e-05], [1.9758876407196743e-05, 1.1105763056005588e-05], [2.19340976058351e-05, 1.15603885523568e-05], [2.4109318804473457e-05, 1.201501404870801e-05], [2.6284540003111814e-05, 1.2469639545059222e-05], [2.845976120175017e-05, 1.2924265041410433e-05], [1.6020641587110248e-05, 1.0146733952173472e-05], [-1.1032818840807956e-05, 4.13704627734834e-06], [-2.347193845544788e-05, 1.35951518811138e-06], [-2.1296717256809523e-05, 1.8141406844625917e-06], [-1.9121496058171166e-05, 2.2687661808138033e-06], [-1.694627485953281e-05, 2.723391677165015e-06], [-1.4771053660894453e-05, 3.1780171735162266e-06], [-1.2595832462256098e-05, 3.6326426698674382e-06], [-1.0420611263617743e-05, 4.08726816621865e-06], [-8.245390064979387e-06, 4.541893662569862e-06], [-6.070168866341032e-06, 4.996519158921074e-06], [-3.8949476677026765e-06, 5.4511446552722865e-06], [-1.7197264690643212e-06, 5.9057701516234985e-06], [4.554947295740342e-07, 6.3603956479747106e-06], [2.6307159282123895e-06, 6.815021144325923e-06], [4.805937126850745e-06, 7.269646640677135e-06], [6.9811583254891e-06, 7.724272137028347e-06], [9.156379524127456e-06, 8.178897633379558e-06], [1.1331600722765811e-05, 8.63352312973077e-06], [1.3506821921404166e-05, 9.08814862608198e-06], [1.568204312004252e-05, 9.542774122433192e-06], [1.7857264318680877e-05, 9.997399618784403e-06], [2.0032485517319234e-05, 1.0452025115135614e-05], [2.220770671595759e-05, 1.0906650611486825e-05], [2.4382927914595948e-05, 1.1361276107838036e-05], [2.6558149113234305e-05, 1.1815901604189248e-05], [2.8733370311872662e-05, 1.2270527100540459e-05], [1.629425069723274e-05, 9.492996011303498e-06], [-1.0759209730685465e-05, 3.483308336478366e-06], [-2.319832934532539e-05, 7.057772472414059e-07], [-2.1023108146687032e-05, 1.1604027435926175e-06], [-1.8847886948048675e-05, 1.6150282399438292e-06], [-1.6672665749410318e-05, 2.069653736295041e-06], [-1.4497444550771962e-05, 2.5242792326462524e-06], [-1.2322223352133607e-05, 2.978904728997464e-06], [-1.0147002153495252e-05, 3.4335302253486757e-06], [-7.971780954856896e-06, 3.888155721699887e-06], [-5.796559756218541e-06, 4.342781218051099e-06], [-3.6213385575801858e-06, 4.7974067144023114e-06], [-1.4461173589418304e-06, 5.2520322107535235e-06], [7.291038396965249e-07, 5.7066577071047356e-06], [2.9043250383348803e-06, 6.161283203455948e-06], [5.079546236973236e-06, 6.61590869980716e-06], [7.254767435611591e-06, 7.070534196158372e-06], [9.429988634249946e-06, 7.525159692509584e-06], [1.1605209832888302e-05, 7.979785188860795e-06], [1.3780431031526657e-05, 8.434410685212006e-06], [1.595565223016501e-05, 8.889036181563217e-06], [1.8130873428803368e-05, 9.343661677914429e-06], [2.0306094627441725e-05, 9.79828717426564e-06], [2.2481315826080082e-05, 1.0252912670616851e-05], [2.465653702471844e-05, 1.0707538166968062e-05], [2.6831758223356796e-05, 1.1162163663319273e-05], [2.9006979421995153e-05, 1.1616789159670485e-05], [1.656785980735523e-05, 8.839258070433524e-06], [-1.0485600620562975e-05, 2.829570395608392e-06], [-2.2924720235202898e-05, 5.2039306371431735e-08], [-2.074949903656454e-05, 5.066648027226435e-07], [-1.8574277837926184e-05, 9.612902990738552e-07], [-1.6399056639287827e-05, 1.415915795425067e-06], [-1.4223835440649472e-05, 1.8705412917762787e-06], [-1.2048614242011116e-05, 2.3251667881274903e-06], [-9.873393043372761e-06, 2.779792284478702e-06], [-7.698171844734406e-06, 3.2344177808299136e-06], [-5.52295064609605e-06, 3.6890432771811252e-06], [-3.347729447457695e-06, 4.143668773532337e-06], [-1.1725082488193397e-06, 4.598294269883549e-06], [1.0027129498190157e-06, 5.052919766234761e-06], [3.177934148457371e-06, 5.5075452625859734e-06], [5.353155347095726e-06, 5.9621707589371855e-06], [7.528376545734082e-06, 6.4167962552883976e-06], [9.703597744372437e-06, 6.87142175163961e-06], [1.1878818943010792e-05, 7.326047247990822e-06], [1.4054040141649148e-05, 7.780672744342034e-06], [1.62292613402875e-05, 8.235298240693245e-06], [1.840448253892586e-05, 8.689923737044456e-06], [2.0579703737564215e-05, 9.144549233395667e-06], [2.2754924936202572e-05, 9.599174729746879e-06], [2.493014613484093e-05, 1.005380022609809e-05], [2.7105367333479287e-05, 1.0508425722449301e-05], [2.9280588532117644e-05, 1.0963051218800512e-05], [1.684146891747772e-05, 8.185520129563552e-06], [-1.0211991510440484e-05, 2.1758324547384194e-06], [-2.2651111125080407e-05, -6.016986344985407e-07], [-2.047588992644205e-05, -1.47073138147329e-07], [-1.8300668727803693e-05, 3.0755235820388274e-07], [-1.6125447529165336e-05, 7.621778545550945e-07], [-1.3950226330526981e-05, 1.2168033509063062e-06], [-1.1775005131888626e-05, 1.6714288472575178e-06], [-9.59978393325027e-06, 2.1260543436087295e-06], [-7.424562734611915e-06, 2.580679839959941e-06], [-5.24934153597356e-06, 3.0353053363111527e-06], [-3.0741203373352043e-06, 3.4899308326623644e-06], [-8.98899138696849e-07, 3.944556329013576e-06], [1.2763220599415064e-06, 4.399181825364788e-06], [3.4515432585798617e-06, 4.853807321716e-06], [5.626764457218217e-06, 5.308432818067212e-06], [7.801985655856572e-06, 5.763058314418424e-06], [9.977206854494928e-06, 6.217683810769636e-06], [1.2152428053133283e-05, 6.672309307120848e-06], [1.4327649251771638e-05, 7.12693480347206e-06], [1.6502870450409992e-05, 7.5815602998232725e-06], [1.867809164904835e-05, 8.036185796174484e-06], [2.0853312847686706e-05, 8.490811292525695e-06], [2.3028534046325063e-05, 8.945436788876906e-06], [2.520375524496342e-05, 9.400062285228117e-06], [2.7378976443601777e-05, 9.854687781579329e-06], [2.9554197642240134e-05, 1.030931327793054e-05], [1.711507802760021e-05, 7.531782188693579e-06], [-9.938382400317993e-06, 1.522094513868447e-06], [-2.2377502014957917e-05, -1.2554365753685132e-06], [-2.020228081631956e-05, -8.008110790173015e-07], [-1.8027059617681203e-05, -3.4618558266608974e-07], [-1.5851838419042846e-05, 1.08439913685122e-07], [-1.367661722040449e-05, 5.630654100363337e-07], [-1.1501396021766135e-05, 1.0176909063875454e-06], [-9.32617482312778e-06, 1.472316402738757e-06], [-7.150953624489424e-06, 1.9269418990899686e-06], [-4.975732425851069e-06, 2.3815673954411803e-06], [-2.8005112272127136e-06, 2.836192891792392e-06], [-6.252900285743582e-07, 3.2908183881436035e-06], [1.5499311700639971e-06, 3.745443884494815e-06], [3.7251523687023525e-06, 4.200069380846027e-06], [5.900373567340708e-06, 4.654694877197239e-06], [8.075594765979063e-06, 5.109320373548451e-06], [1.0250815964617418e-05, 5.563945869899663e-06], [1.2426037163255774e-05, 6.018571366250875e-06], [1.460125836189413e-05, 6.473196862602087e-06], [1.6776479560532483e-05, 6.927822358953299e-06], [1.895170075917084e-05, 7.382447855304511e-06], [2.1126921957809197e-05, 7.837073351655722e-06], [2.3302143156447554e-05, 8.291698848006934e-06], [2.547736435508591e-05, 8.746324344358145e-06], [2.7652585553724268e-05, 9.200949840709356e-06], [2.9827806752362625e-05, 9.655575337060567e-06], [1.73886871377227e-05, 6.878044247823607e-06], [-9.664773290195502e-06, 8.683565729984744e-07], [-2.2103892904835426e-05, -1.9091745162384857e-06], [-1.992867170619707e-05, -1.454549019887274e-06], [-1.7753450507558712e-05, -9.999235235360624e-07], [-1.5578229308920355e-05, -5.452980271848507e-07], [-1.3403008110282e-05, -9.067253083363894e-08], [-1.1227786911643644e-05, 3.639529655175728e-07], [-9.052565713005289e-06, 8.185784618687845e-07], [-6.8773445143669335e-06, 1.2732039582199962e-06], [-4.702123315728578e-06, 1.7278294545712078e-06], [-2.526902117090223e-06, 2.1824549509224194e-06], [-3.516809184518675e-07, 2.637080447273631e-06], [1.8235402801864878e-06, 3.0917059436248427e-06], [3.998761478824843e-06, 3.5463314399760543e-06], [6.1739826774631985e-06, 4.000956936327266e-06], [8.349203876101554e-06, 4.4555824326784784e-06], [1.052442507473991e-05, 4.9102079290296905e-06], [1.2699646273378265e-05, 5.3648334253809026e-06], [1.487486747201662e-05, 5.819458921732115e-06], [1.7050088670654974e-05, 6.274084418083327e-06], [1.922530986929333e-05, 6.728709914434539e-06], [2.1400531067931688e-05, 7.183335410785751e-06], [2.3575752266570045e-05, 7.637960907136963e-06], [2.57509734652084e-05, 8.092586403488174e-06], [2.792619466384676e-05, 8.547211899839385e-06], [3.0101415862485116e-05, 9.001837396190596e-06], [1.7662296247845192e-05, 6.224306306953636e-06], [-9.391164180073012e-06, 2.1461863212850365e-07], [-2.1830283794712935e-05, -2.5629124571084565e-06], [-1.9655062596074578e-05, -2.108286960757245e-06], [-1.747984139743622e-05, -1.6536614644060332e-06], [-1.5304620198797864e-05, -1.1990359680548216e-06], [-1.3129399000159509e-05, -7.444104717036098e-07], [-1.0954177801521153e-05, -2.897849753523981e-07], [-8.778956602882798e-06, 1.6484052099881365e-07], [-6.603735404244443e-06, 6.194660173500254e-07], [-4.4285142056060874e-06, 1.074091513701237e-06], [-2.253293006967732e-06, 1.5287170100524487e-06], [-7.807180832937676e-08, 1.9833425064036603e-06], [2.0971493903089786e-06, 2.437968002754872e-06], [4.272370588947334e-06, 2.8925934991060835e-06], [6.447591787585689e-06, 3.347218995457295e-06], [8.622812986224045e-06, 3.801844491808507e-06], [1.07980341848624e-05, 4.256469988159719e-06], [1.2973255383500755e-05, 4.711095484510931e-06], [1.514847658213911e-05, 5.165720980862143e-06], [1.7323697780777464e-05, 5.620346477213355e-06], [1.949891897941582e-05, 6.074971973564567e-06], [2.167414017805418e-05, 6.529597469915779e-06], [2.3849361376692535e-05, 6.984222966266991e-06], [2.6024582575330892e-05, 7.438848462618203e-06], [2.819980377396925e-05, 7.893473958969414e-06], [3.0375024972607606e-05, 8.348099455320626e-06], [1.7935905357967683e-05, 5.570568366083665e-06], [-9.117555069950521e-06, -4.3911930874146713e-07], [-2.1556674684590445e-05, -3.2166503979784272e-06], [-1.9381453485952087e-05, -2.7620249016272156e-06], [-1.720623228731373e-05, -2.307399405276004e-06], [-1.5031011088675375e-05, -1.8527739089247923e-06], [-1.285578989003702e-05, -1.3981484125735807e-06], [-1.0680568691398664e-05, -9.43522916222369e-07], [-8.505347492760309e-06, -4.888974198711572e-07], [-6.330126294121954e-06, -3.42719235199455e-08], [-4.154905095483598e-06, 4.2035357283126624e-07], [-1.979683896845243e-06, 8.74979069182478e-07], [1.9553730179311228e-07, 1.3296045655336897e-06], [2.3707585004314676e-06, 1.7842300618849016e-06], [4.545979699069823e-06, 2.238855558236113e-06], [6.721200897708178e-06, 2.693481054587325e-06], [8.896422096346534e-06, 3.1481065509385365e-06], [1.1071643294984889e-05, 3.602732047289748e-06], [1.3246864493623244e-05, 4.05735754364096e-06], [1.5422085692261598e-05, 4.511983039992172e-06], [1.7597306890899955e-05, 4.966608536343384e-06], [1.9772528089538312e-05, 5.421234032694596e-06], [2.194774928817667e-05, 5.875859529045808e-06], [2.4122970486815026e-05, 6.3304850253970204e-06], [2.6298191685453383e-05, 6.7851105217482325e-06], [2.847341288409174e-05, 7.2397360180994445e-06], [3.06486340827301e-05, 7.694361514450657e-06], [1.8209514468090174e-05, 4.916830425213696e-06], [-8.84394595982803e-06, -1.0928572496114362e-06], [-2.1283065574467954e-05, -3.870388338848397e-06], [-1.9107844375829597e-05, -3.415762842497185e-06], [-1.693262317719124e-05, -2.9611373461459735e-06], [-1.4757401978552884e-05, -2.506511849794762e-06], [-1.2582180779914529e-05, -2.0518863534435502e-06], [-1.0406959581276174e-05, -1.5972608570923386e-06], [-8.231738382637818e-06, -1.142635360741127e-06], [-6.056517183999463e-06, -6.880098643899152e-07], [-3.881295985361108e-06, -2.3338436803870348e-07], [-1.7060747867227523e-06, 2.2124112831250826e-07], [4.69146411915603e-07, 6.7586662466372e-07], [2.6443676105539583e-06, 1.1304921210149316e-06], [4.819588809192314e-06, 1.5851176173661433e-06], [6.994810007830669e-06, 2.039743113717355e-06], [9.170031206469024e-06, 2.4943686100685665e-06], [1.134525240510738e-05, 2.948994106419778e-06], [1.3520473603745735e-05, 3.40361960277099e-06], [1.569569480238409e-05, 3.858245099122201e-06], [1.7870916001022446e-05, 4.3128705954734135e-06], [2.0046137199660803e-05, 4.7674960918246255e-06], [2.222135839829916e-05, 5.222121588175838e-06], [2.4396579596937517e-05, 5.67674708452705e-06], [2.6571800795575874e-05, 6.131372580878262e-06], [2.874702199421423e-05, 6.585998077229474e-06], [3.092224319285259e-05, 7.040623573580686e-06], [1.8483123578212664e-05, 4.263092484343725e-06], [-8.57033684970554e-06, -1.746595190481407e-06], [-2.1009456464345463e-05, -4.5241262797183675e-06], [-1.8834235265707106e-05, -4.0695007833671555e-06], [-1.665901406706875e-05, -3.614875287015944e-06], [-1.4483792868430394e-05, -3.160249790664732e-06], [-1.2308571669792038e-05, -2.7056242943135206e-06], [-1.0133350471153683e-05, -2.250998797962309e-06], [-7.958129272515328e-06, -1.7963733016110973e-06], [-5.782908073876972e-06, -1.3417478052598857e-06], [-3.607686875238617e-06, -8.871223089086739e-07], [-1.4324656766002616e-06, -4.324968125574622e-07], [7.427555220380937e-07, 2.2128683793749533e-08], [2.917976720676449e-06, 4.7675418014496127e-07], [5.093197919314804e-06, 9.31379676496173e-07], [7.26841911795316e-06, 1.3860051728473847e-06], [9.443640316591515e-06, 1.8406306691985966e-06], [1.161886151522987e-05, 2.2952561655498082e-06], [1.3794082713868226e-05, 2.74988166190102e-06], [1.596930391250658e-05, 3.2045071582522315e-06], [1.8144525111144936e-05, 3.659132654603443e-06], [2.0319746309783293e-05, 4.113758150954655e-06], [2.249496750842165e-05, 4.568383647305867e-06], [2.4670188707060008e-05, 5.023009143657079e-06], [2.6845409905698365e-05, 5.477634640008291e-06], [2.902063110433672e-05, 5.932260136359503e-06], [3.119585230297508e-05, 6.386885632710715e-06], [1.8756732688335155e-05, 3.6093545434737545e-06], [-8.296727739583049e-06, -2.4003331313513778e-06], [-2.0735847354222972e-05, -5.177864220588338e-06], [-1.8560626155584615e-05, -4.723238724237126e-06], [-1.6385404956946258e-05, -4.268613227885914e-06], [-1.4210183758307903e-05, -3.8139877315347026e-06], [-1.2034962559669548e-05, -3.359362235183491e-06], [-9.859741361031192e-06, -2.9047367388322793e-06], [-7.684520162392837e-06, -2.4501112424810677e-06], [-5.5092989637544815e-06, -1.995485746129856e-06], [-3.334077765116126e-06, -1.5408602497786444e-06], [-1.1588565664777709e-06, -1.0862347534274328e-06], [1.0163646321605845e-06, -6.31609257076221e-07], [3.19158583079894e-06, -1.769837607250093e-07], [5.366807029437295e-06, 2.7764173562620244e-07], [7.5420282280756505e-06, 7.322672319774142e-07], [9.717249426714006e-06, 1.1868927283286258e-06], [1.1892470625352361e-05, 1.6415182246798374e-06], [1.4067691823990717e-05, 2.096143721031049e-06], [1.624291302262907e-05, 2.5507692173822607e-06], [1.8418134221267427e-05, 3.0053947137334723e-06], [2.0593355419905784e-05, 3.460020210084684e-06], [2.276857661854414e-05, 3.914645706435896e-06], [2.4943797817182498e-05, 4.369271202787108e-06], [2.7119019015820855e-05, 4.82389669913832e-06], [2.9294240214459212e-05, 5.278522195489532e-06], [3.146946141309757e-05, 5.733147691840744e-06], [1.9030341798457646e-05, 2.9556166026037837e-06], [-8.023118629460558e-06, -3.0540710722213486e-06], [-2.046223824410048e-05, -5.831602161458309e-06], [-1.8287017045462125e-05, -5.376976665107097e-06], [-1.6111795846823768e-05, -4.922351168755885e-06], [-1.3936574648185412e-05, -4.467725672404673e-06], [-1.1761353449547057e-05, -4.013100176053461e-06], [-9.586132250908701e-06, -3.5584746797022492e-06], [-7.410911052270346e-06, -3.1038491833510376e-06], [-5.235689853631991e-06, -2.649223686999826e-06], [-3.0604686549936355e-06, -2.1945981906486143e-06], [-8.852474563552801e-07, -1.7399726942974027e-06], [1.2899737422830752e-06, -1.285347197946191e-06], [3.4651949409214305e-06, -8.307217015949793e-07], [5.640416139559786e-06, -3.760962052437676e-07], [7.815637338198141e-06, 7.852929110744414e-08], [9.990858536836497e-06, 5.331547874586559e-07], [1.2166079735474852e-05, 9.877802838098675e-07], [1.4341300934113207e-05, 1.4424057801610791e-06], [1.651652213275156e-05, 1.8970312765122908e-06], [1.8691743331389918e-05, 2.3516567728635024e-06], [2.0866964530028275e-05, 2.806282269214714e-06], [2.3042185728666632e-05, 3.2609077655659257e-06], [2.521740692730499e-05, 3.7155332619171373e-06], [2.7392628125943346e-05, 4.170158758268349e-06], [2.9567849324581703e-05, 4.624784254619561e-06], [3.174307052322006e-05, 5.0794097509707735e-06], [1.9303950908580137e-05, 2.301878661733813e-06], [-7.749509519338067e-06, -3.7078090130913193e-06], [-2.018862913397799e-05, -6.48534010232828e-06], [-1.8013407935339634e-05, -6.030714605977068e-06], [-1.5838186736701277e-05, -5.576089109625856e-06], [-1.3662965538062921e-05, -5.121463613274644e-06], [-1.1487744339424566e-05, -4.666838116923432e-06], [-9.31252314078621e-06, -4.21221262057222e-06], [-7.137301942147855e-06, -3.757587124221008e-06], [-4.9620807435095e-06, -3.3029616278697963e-06], [-2.7868595448711447e-06, -2.8483361315185847e-06], [-6.116383462327894e-07, -2.393710635167373e-06], [1.563582852405566e-06, -1.9390851388161614e-06], [3.7388040510439213e-06, -1.4844596424649498e-06], [5.914025249682277e-06, -1.0298341461137382e-06], [8.089246448320632e-06, -5.752086497625264e-07], [1.0264467646958987e-05, -1.205831534113147e-07], [1.2439688845597343e-05, 3.3404234293989705e-07], [1.4614910044235698e-05, 7.886678392911088e-07], [1.679013124287405e-05, 1.2432933356423204e-06], [1.896535244151241e-05, 1.697918831993532e-06], [2.1140573640150766e-05, 2.1525443283447437e-06], [2.3315794838789123e-05, 2.6071698246959553e-06], [2.549101603742748e-05, 3.061795321047167e-06], [2.7666237236065837e-05, 3.5164208173983786e-06], [2.9841458434704194e-05, 3.971046313749591e-06], [3.201667963334255e-05, 4.425671810100803e-06], [1.9577560018702627e-05, 1.6481407208638422e-06], [-7.475900409215577e-06, -4.36154695396129e-06], [-1.99150200238555e-05, -7.139078043198251e-06], [-1.7739798825217143e-05, -6.684452546847039e-06], [-1.5564577626578786e-05, -6.2298270504958265e-06], [-1.338935642794043e-05, -5.7752015541446145e-06], [-1.1214135229302075e-05, -5.3205760577934024e-06], [-9.03891403066372e-06, -4.86595056144219e-06], [-6.863692832025365e-06, -4.411325065090978e-06], [-4.688471633387009e-06, -3.956699568739766e-06], [-2.513250434748654e-06, -3.5020740723885546e-06], [-3.3802923611029867e-07, -3.047448576037343e-06], [1.8371919625280567e-06, -2.5928230796861314e-06], [4.012413161166412e-06, -2.1381975833349197e-06], [6.187634359804767e-06, -1.683572086983708e-06], [8.362855558443123e-06, -1.2289465906324965e-06], [1.0538076757081478e-05, -7.743210942812847e-07], [1.2713297955719833e-05, -3.19695597930073e-07], [1.4888519154358189e-05, 1.3492989842113875e-07], [1.7063740352996542e-05, 5.895553947723505e-07], [1.92389615516349e-05, 1.0441808911235621e-06], [2.1414182750273256e-05, 1.4988063874747738e-06], [2.3589403948911613e-05, 1.9534318838259854e-06], [2.576462514754997e-05, 2.408057380177197e-06], [2.7939846346188328e-05, 2.8626828765284087e-06], [3.0115067544826685e-05, 3.3173083728796203e-06], [3.229028874346504e-05, 3.771933869230832e-06], [1.9851169128825118e-05, 9.944027799938714e-07], [-7.202291299093086e-06, -5.015284894831261e-06], [-1.964141091373301e-05, -7.792815984068221e-06], [-1.7466189715094652e-05, -7.338190487717009e-06], [-1.5290968516456295e-05, -6.883564991365797e-06], [-1.311574731781794e-05, -6.428939495014585e-06], [-1.0940526119179585e-05, -5.974313998663373e-06], [-8.76530492054123e-06, -5.519688502312161e-06], [-6.590083721902874e-06, -5.065063005960949e-06], [-4.414862523264519e-06, -4.610437509609737e-06], [-2.2396413246261633e-06, -4.155812013258525e-06], [-6.442012598780794e-08, -3.7011865169073133e-06], [2.1108010726505474e-06, -3.2465610205561017e-06], [4.286022271288903e-06, -2.79193552420489e-06], [6.461243469927258e-06, -2.3373100278536785e-06], [8.636464668565613e-06, -1.8826845315024668e-06], [1.0811685867203969e-05, -1.4280590351512552e-06], [1.2986907065842324e-05, -9.734335388000436e-07], [1.516212826448068e-05, -5.188080424488318e-07], [1.7337349463119033e-05, -6.418254609762008e-08], [1.951257066175739e-05, 3.9044295025359166e-07], [2.1687791860395747e-05, 8.450684466048034e-07], [2.3863013059034104e-05, 1.299693942956015e-06], [2.603823425767246e-05, 1.7543194393072267e-06], [2.8213455456310818e-05, 2.2089449356584383e-06], [3.0388676654949175e-05, 2.66357043200965e-06], [3.256389785358753e-05, 3.1181959283608616e-06], [2.012477823894761e-05, 3.4066483912390103e-07], [-6.928682188970595e-06, -5.669022835701232e-06], [-1.936780180361052e-05, -8.446553924938192e-06], [-1.719258060497216e-05, -7.991928428586981e-06], [-1.5017359406333806e-05, -7.537302932235769e-06], [-1.2842138207695451e-05, -7.082677435884557e-06], [-1.0666917009057096e-05, -6.628051939533345e-06], [-8.49169581041874e-06, -6.173426443182133e-06], [-6.316474611780385e-06, -5.718800946830921e-06], [-4.14125341314203e-06, -5.264175450479709e-06], [-1.9660322145036742e-06, -4.809549954128497e-06], [2.091889841346811e-07, -4.3549244577772846e-06], [2.3844101827730364e-06, -3.9002989614260725e-06], [4.559631381411392e-06, -3.445673465074861e-06], [6.734852580049747e-06, -2.9910479687236492e-06], [8.910073778688102e-06, -2.5364224723724376e-06], [1.1085294977326458e-05, -2.081796976021226e-06], [1.3260516175964813e-05, -1.6271714796700143e-06], [1.5435737374603167e-05, -1.1725459833188027e-06], [1.7610958573241524e-05, -7.17920486967591e-07], [1.978617977187988e-05, -2.632949906163792e-07], [2.1961400970518238e-05, 1.9133050573483251e-07], [2.4136622169156595e-05, 6.459560020860443e-07], [2.6311843367794952e-05, 1.1005814984372559e-06], [2.848706456643331e-05, 1.5552069947884675e-06], [3.0662285765071666e-05, 2.009832491139679e-06], [3.283750696371002e-05, 2.4644579874908908e-06], [2.03983873490701e-05, -3.1307310174606975e-07], [-6.6550730788481044e-06, -6.3227607765712025e-06], [-1.9094192693488028e-05, -9.100291865808163e-06], [-1.691897149484967e-05, -8.645666369456952e-06], [-1.4743750296211316e-05, -8.19104087310574e-06], [-1.256852909757296e-05, -7.73641537675453e-06], [-1.0393307898934605e-05, -7.281789880403317e-06], [-8.21808670029625e-06, -6.827164384052105e-06], [-6.042865501657894e-06, -6.372538887700893e-06], [-3.867644303019539e-06, -5.917913391349681e-06], [-1.6924231043811835e-06, -5.463287894998469e-06], [4.827980942571718e-07, -5.008662398647257e-06], [2.658019292895527e-06, -4.554036902296045e-06], [4.8332404915338825e-06, -4.099411405944833e-06], [7.008461690172238e-06, -3.6447859095936213e-06], [9.183682888810593e-06, -3.1901604132424096e-06], [1.1358904087448949e-05, -2.735534916891198e-06], [1.3534125286087304e-05, -2.2809094205399864e-06], [1.5709346484725658e-05, -1.8262839241887748e-06], [1.7884567683364015e-05, -1.3716584278375631e-06], [2.005978888200237e-05, -9.170329314863514e-07], [2.223501008064073e-05, -4.6240743513513964e-07], [2.4410231279279086e-05, -7.781938783927904e-09], [2.6585452477917443e-05, 4.4684355756728383e-07], [2.87606736765558e-05, 9.014690539184956e-07], [3.093589487519416e-05, 1.3560945502697073e-06], [3.3111116073832514e-05, 1.8107200466209192e-06], [2.067199645919259e-05, -9.668110426160414e-07], [-6.381463968725614e-06, -6.976498717441173e-06], [-1.8820583583365537e-05, -9.754029806678134e-06], [-1.664536238472718e-05, -9.299404310326923e-06], [-1.4470141186088825e-05, -8.844778813975711e-06], [-1.229491998745047e-05, -8.3901533176245e-06], [-1.0119698788812114e-05, -7.935527821273289e-06], [-7.944477590173759e-06, -7.480902324922077e-06], [-5.7692563915354035e-06, -7.026276828570865e-06], [-3.594035192897048e-06, -6.571651332219653e-06], [-1.4188139942586928e-06, -6.117025835868441e-06], [7.564072043796626e-07, -5.662400339517229e-06], [2.931628403018018e-06, -5.207774843166017e-06], [5.106849601656373e-06, -4.7531493468148045e-06], [7.282070800294729e-06, -4.2985238504635925e-06], [9.457291998933084e-06, -3.8438983541123804e-06], [1.163251319757144e-05, -3.389272857761169e-06], [1.3807734396209795e-05, -2.934647361409957e-06], [1.5982955594848148e-05, -2.4800218650587455e-06], [1.8158176793486505e-05, -2.025396368707534e-06], [2.0333397992124862e-05, -1.5707708723563223e-06], [2.250861919076322e-05, -1.1161453760051106e-06], [2.4683840389401576e-05, -6.615198796538989e-07], [2.6859061588039933e-05, -2.0689438330268716e-07], [2.903428278667829e-05, 2.477311130485246e-07], [3.120950398531665e-05, 7.023566093997363e-07], [3.3384725183955005e-05, 1.156982105750948e-06], [2.094560556931508e-05, -1.6205489834860126e-06], [-6.107854858603123e-06, -7.630236658311146e-06], [-1.8546974473243046e-05, -1.0407767747548106e-05], [-1.637175327460469e-05, -9.953142251196895e-06], [-1.4196532075966334e-05, -9.498516754845684e-06], [-1.2021310877327979e-05, -9.043891258494473e-06], [-9.846089678689623e-06, -8.589265762143261e-06], [-7.670868480051268e-06, -8.13464026579205e-06], [-5.495647281412913e-06, -7.680014769440839e-06], [-3.3204260827745574e-06, -7.225389273089627e-06], [-1.145204884136202e-06, -6.770763776738415e-06], [1.0300163145021533e-06, -6.316138280387203e-06], [3.2052375131405086e-06, -5.861512784035991e-06], [5.380458711778864e-06, -5.406887287684779e-06], [7.555679910417219e-06, -4.952261791333567e-06], [9.730901109055575e-06, -4.497636294982355e-06], [1.190612230769393e-05, -4.0430107986311425e-06], [1.4081343506332285e-05, -3.588385302279931e-06], [1.625656470497064e-05, -3.1337598059287193e-06], [1.8431785903608996e-05, -2.6791343095775076e-06], [2.0607007102247353e-05, -2.224508813226296e-06], [2.278222830088571e-05, -1.7698833168750844e-06], [2.4957449499524067e-05, -1.3152578205238727e-06], [2.7132670698162424e-05, -8.60632324172661e-07], [2.930789189680078e-05, -4.0600682782144927e-07], [3.148311309543914e-05, 4.861866852976247e-08], [3.3658334294077495e-05, 5.032441648809742e-07], [2.1219214679437572e-05, -2.2742869243559863e-06], [-5.834245748480632e-06, -8.283974599181118e-06], [-1.8273365363120556e-05, -1.1061505688418079e-05], [-1.60981441644822e-05, -1.0606880192066868e-05], [-1.3922922965843843e-05, -1.0152254695715656e-05], [-1.1747701767205488e-05, -9.697629199364445e-06], [-9.572480568567133e-06, -9.243003703013234e-06], [-7.397259369928777e-06, -8.788378206662023e-06], [-5.222038171290422e-06, -8.333752710310811e-06], [-3.0468169726520667e-06, -7.8791272139596e-06], [-8.715957740137113e-07, -7.424501717608388e-06], [1.303625424624644e-06, -6.969876221257176e-06], [3.4788466232629994e-06, -6.515250724905964e-06], [5.654067821901355e-06, -6.060625228554752e-06], [7.82928902053971e-06, -5.60599973220354e-06], [1.0004510219178065e-05, -5.151374235852328e-06], [1.217973141781642e-05, -4.696748739501116e-06], [1.4354952616454776e-05, -4.242123243149904e-06], [1.653017381509313e-05, -3.787497746798692e-06], [1.8705395013731487e-05, -3.3328722504474805e-06], [2.0880616212369844e-05, -2.878246754096269e-06], [2.30558374110082e-05, -2.4236212577450573e-06], [2.5231058609646558e-05, -1.9689957613938456e-06], [2.7406279808284915e-05, -1.514370265042634e-06], [2.9581501006923272e-05, -1.0597447686914224e-06], [3.175672220556163e-05, -6.051192723402106e-07], [3.3931943404199986e-05, -1.504937759889989e-07], [2.1492823789560062e-05, -2.9280248652259592e-06], [-5.5606366383581415e-06, -8.93771254005109e-06], [-1.7999756252998065e-05, -1.1715243629288051e-05], [-1.5824535054359708e-05, -1.126061813293684e-05], [-1.3649313855721353e-05, -1.0805992636585629e-05], [-1.1474092657082997e-05, -1.0351367140234418e-05], [-9.298871458444642e-06, -9.896741643883206e-06], [-7.123650259806287e-06, -9.442116147531995e-06], [-4.948429061167931e-06, -8.987490651180784e-06], [-2.773207862529576e-06, -8.532865154829573e-06], [-5.979866638912206e-07, -8.078239658478362e-06], [1.5772345347471348e-06, -7.6236141621271495e-06], [3.75245573338549e-06, -7.168988665775937e-06], [5.9276769320238454e-06, -6.714363169424725e-06], [8.1028981306622e-06, -6.259737673073513e-06], [1.0278119329300556e-05, -5.805112176722301e-06], [1.2453340527938911e-05, -5.350486680371089e-06], [1.4628561726577267e-05, -4.895861184019877e-06], [1.680378292521562e-05, -4.441235687668665e-06], [1.8979004123853977e-05, -3.986610191317453e-06], [2.1154225322492335e-05, -3.5319846949662414e-06], [2.332944652113069e-05, -3.0773591986150297e-06], [2.550466771976905e-05, -2.622733702263818e-06], [2.7679888918407406e-05, -2.1681082059126065e-06], [2.9855110117045763e-05, -1.7134827095613949e-06], [3.203033131568412e-05, -1.2588572132101832e-06], [3.420555251432248e-05, -8.042317168589715e-07], [2.1766432899682553e-05, -3.581762806095932e-06], [-5.287027528235651e-06, -9.591450480921065e-06], [-1.7726147142875574e-05, -1.2368981570158025e-05], [-1.5550925944237217e-05, -1.1914356073806814e-05], [-1.3375704745598862e-05, -1.1459730577455603e-05], [-1.1200483546960507e-05, -1.1005105081104392e-05], [-9.025262348322151e-06, -1.055047958475318e-05], [-6.850041149683796e-06, -1.009585408840197e-05], [-4.6748199510454405e-06, -9.641228592050758e-06], [-2.499598752407085e-06, -9.186603095699547e-06], [-3.2437755376872985e-07, -8.731977599348336e-06], [1.8508436448696255e-06, -8.277352102997124e-06], [4.026064843507981e-06, -7.822726606645913e-06], [6.201286042146336e-06, -7.368101110294701e-06], [8.376507240784692e-06, -6.913475613943489e-06], [1.0551728439423047e-05, -6.458850117592277e-06], [1.2726949638061402e-05, -6.004224621241065e-06], [1.4902170836699758e-05, -5.549599124889853e-06], [1.707739203533811e-05, -5.094973628538641e-06], [1.9252613233976468e-05, -4.640348132187429e-06], [2.1427834432614825e-05, -4.185722635836217e-06], [2.3603055631253182e-05, -3.731097139485005e-06], [2.577827682989154e-05, -3.2764716431337936e-06], [2.7953498028529896e-05, -2.821846146782582e-06], [3.0128719227168253e-05, -2.3672206504313703e-06], [3.230394042580661e-05, -1.9125951540801587e-06], [3.447916162444497e-05, -1.457969657728947e-06], [2.2040042009805044e-05, -4.2355007469659076e-06], [-5.01341841811316e-06, -1.0245188421791039e-05], [-1.7452538032753084e-05, -1.3022719511028e-05], [-1.5277316834114726e-05, -1.2568094014676788e-05], [-1.3102095635476371e-05, -1.2113468518325577e-05], [-1.0926874436838016e-05, -1.1658843021974366e-05], [-8.75165323819966e-06, -1.1204217525623155e-05], [-6.576432039561305e-06, -1.0749592029271943e-05], [-4.40121084092295e-06, -1.0294966532920732e-05], [-2.2259896422845945e-06, -9.840341036569521e-06], [-5.0768443646239116e-08, -9.38571554021831e-06], [2.1244527549921162e-06, -8.931090043867099e-06], [4.2996739536304716e-06, -8.476464547515887e-06], [6.474895152268827e-06, -8.021839051164676e-06], [8.650116350907182e-06, -7.567213554813464e-06], [1.0825337549545538e-05, -7.112588058462252e-06], [1.3000558748183893e-05, -6.65796256211104e-06], [1.5175779946822248e-05, -6.203337065759828e-06], [1.7351001145460602e-05, -5.748711569408616e-06], [1.952622234409896e-05, -5.294086073057404e-06], [2.1701443542737316e-05, -4.839460576706192e-06], [2.3876664741375673e-05, -4.38483508035498e-06], [2.605188594001403e-05, -3.930209584003768e-06], [2.8227107138652387e-05, -3.475584087652556e-06], [3.0402328337290744e-05, -3.0209585913013445e-06], [3.25775495359291e-05, -2.566333094950133e-06], [3.475277073456746e-05, -2.111707598598921e-06], [2.2313651119927535e-05, -4.889238687835882e-06], [-4.739809307990669e-06, -1.0898926362661015e-05], [-1.7178928922630593e-05, -1.3676457451897975e-05], [-1.5003707723992237e-05, -1.3221831955546764e-05], [-1.2828486525353882e-05, -1.2767206459195553e-05], [-1.0653265326715527e-05, -1.2312580962844342e-05], [-8.478044128077171e-06, -1.185795546649313e-05], [-6.302822929438816e-06, -1.140332997014192e-05], [-4.127601730800461e-06, -1.0948704473790708e-05], [-1.9523805321621054e-06, -1.0494078977439497e-05], [2.2284066647624992e-07, -1.0039453481088286e-05], [2.3980618651146053e-06, -9.584827984737075e-06], [4.573283063752961e-06, -9.130202488385863e-06], [6.748504262391316e-06, -8.675576992034652e-06], [8.923725461029671e-06, -8.220951495683441e-06], [1.1098946659668027e-05, -7.76632599933223e-06], [1.3274167858306382e-05, -7.311700502981018e-06], [1.5449389056944736e-05, -6.8570750066298056e-06], [1.7624610255583093e-05, -6.4024495102785935e-06], [1.979983145422145e-05, -5.9478240139273814e-06], [2.1975052652859807e-05, -5.493198517576169e-06], [2.4150273851498164e-05, -5.038573021224957e-06], [2.632549505013652e-05, -4.583947524873745e-06], [2.8500716248774878e-05, -4.129322028522533e-06], [3.0675937447413235e-05, -3.6746965321713216e-06]]
  in  "Aktiv":T1(array[ring])=[enum."GalvoX", enum."GalvoY"]
  out "Galvo too far":cluster{"x":dbl, "y":dbl}={"x"=1.087610599319179e-06, "y"=2.2731274817560613e-07}
  out "Galvo too late time":dbl=5.000000000000006e-06
  out "min Line+turn":dbl=0.000246633054887395
  out "exactTurn [s]":dbl=4.500000000000001e-05 format="%_6g"
  out "AD/pixel":u32=9
  out "Pixeltime":dbl=2.25e-06
  out "TotalPixel":u32=120
  out "validTotalCycles":u32=27
  out "ini":T2={"Bitsize-Zwischenbild"=5.5926e-07, "CCDmin"=7850.0, "CCDscale"=-10.85, "GalvoCycle"=1.2e-05, "Ext.AD-clock"=4000000.0, "Steps per optical density"=53.33} {"CCDscale" format="%.2f"; "CCDmin" format="%.2f"; "Bitsize-Zwischenbild" format="%.2e"}
  out "Zeit [s]/zeile":dbl=0.000225 min=0.0005 step=0.001 format="%^#_6g"
  out "min Galvocycles":u16=25
  # "Used Units: Pixels or meters in the intermediate image\nchanged May 18 2011\nTurn is extended until Pixel-clock is synchronous with GalvoClock\nuses the IncInc (aceleration) feature"
  # "looses 1 cycle as IncInc is changed at lineend and effect is 2 points later! (Inc is 1 later (next))\nneeds some clean up!"
  # "TriggerPin0: During Turn: High (Line End)\nTriggerPin1: During Frame: High (Frame Start)"
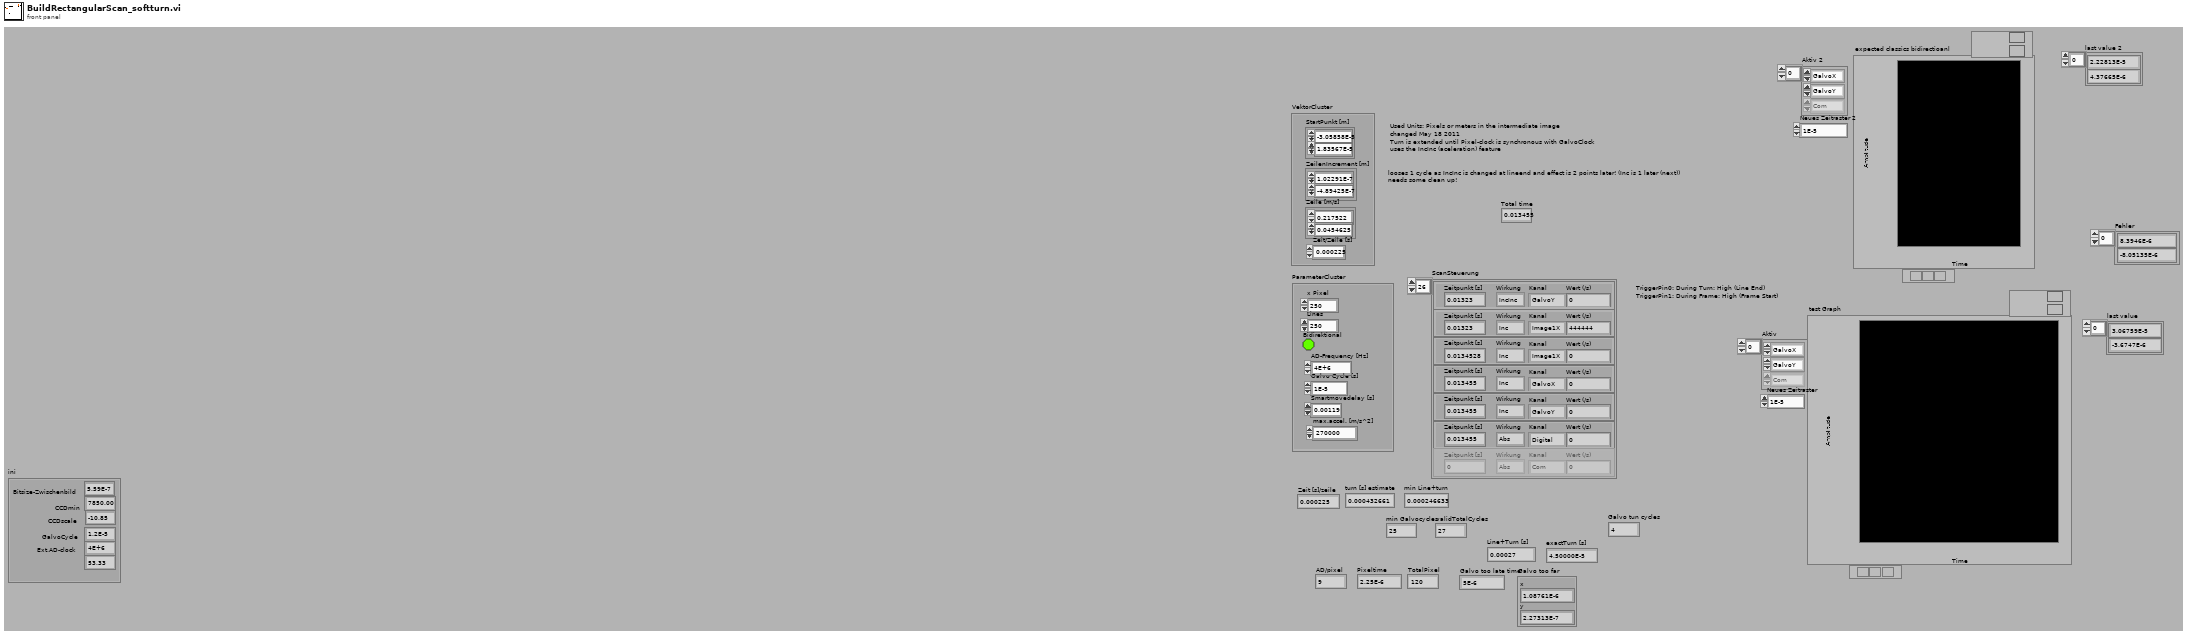
[diagram p1: front panel]
types:
  T1 = enum16{"Com", "AnalogConfig", "AnalogValue", "GalvoX", "GalvoY", "Galvo3", "Galvo4", "Digital", "Free", "Loop", "SMoveTime", "Image1X", "Image1Y", "Image2X", "Image2Y"}[]
  T2 = cluster{"Bitsize-Zwischenbild":dbl, "CCDmin":dbl, "CCDscale":dbl, "GalvoCycle":dbl, "Ext.AD-clock":dbl, "Steps per optical density":dbl}
  T3 = cluster{"StartPunkt [m]":cluster{"x":dbl, "y":dbl}, "ZeilenIncrement [m]":cluster{"x":dbl, "y":dbl}, "Zeile [m/s]":cluster{"x":dbl, "y":dbl}, "Zeit/Zeile [s]":dbl}
  T4 = cluster{"Zeitpunkt [s]":dbl, "Wirkung":enum16{"Abs", "Rel", "Inc", "IncInc", "LoopStart", "LoopEnd"}, "Kanal":enum16{"Com", "AnalogConfig", "AnalogValue", "GalvoX", "GalvoY", "Galvo3", "Galvo4", "Digital", "Free", "Loop", "SMoveTime", "Image1X", "Image1Y", "Image2X", "Image2Y"}, "Wert (/s)":dbl}[]
  T5 = cluster{"x Pixel":i32, "Lines":i32, "Bidirektional":bool, "AD-Frequency [Hz]":dbl, "Galvo Cycle [s]":dbl, "Smartmovedelay [s]":dbl, "max.accel. [m/s^2]":dbl}
  T6 = enum16{"Com", "AnalogConfig", "AnalogValue", "GalvoX", "GalvoY", "Galvo3", "Galvo4", "Digital", "Free", "Loop", "SMoveTime", "Image1X", "Image1Y", "Image2X", "Image2Y"}
  T7 = enum16{"Abs", "Rel", "Inc", "IncInc", "LoopStart", "LoopEnd"}
  T8 = typedef "ScanControl.ctl" = cluster{"Time [s]":dbl, "action":T9, "channel":T10, "value (/s)":dbl}[]
  T9 = typedef "ScanControl_Action.ctl" = enum16{"Abs", "Rel", "Inc", "IncInc", "LoopStart", "LoopEnd", "WaitTriggerRising"}
  T10 = typedef "ScanControl_Channel.ctl" = enum16{"Com", "AnalogConfig", "AnalogValue", "GalvoX", "GalvoY", "Galvo3", "Galvo4", "Digital", "Free", "Loop", "SMoveTime", "Image1X", "Image1Y", "Image2X", "Image2Y"}
  T11 = cluster{"Ende [s] AD+g raster":dbl, "Wirkung":enum16{"Abs", "Rel", "Inc", "IncInc", "LoopStart", "LoopEnd"}, "Kanal":enum16{"Com", "AnalogConfig", "AnalogValue", "GalvoX", "GalvoY", "Galvo3", "Galvo4", "Digital", "Free", "Loop", "SMoveTime", "Image1X", "Image1Y", "Image2X", "Image2Y"}, dbl}
  T12 = cluster{dbl, "Wirkung":enum16{"Abs", "Rel", "Inc", "IncInc", "LoopStart", "LoopEnd"}, "Kanal":enum16{"Com", "AnalogConfig", "AnalogValue", "GalvoX", "GalvoY", "Galvo3", "Galvo4", "Digital", "Free", "Loop", "SMoveTime", "Image1X", "Image1Y", "Image2X", "Image2Y"}, u8}
  T13 = cluster{dbl, "Wirkung":enum16{"Abs", "Rel", "Inc", "IncInc", "LoopStart", "LoopEnd"}, "Kanal":enum16{"Com", "AnalogConfig", "AnalogValue", "GalvoX", "GalvoY", "Galvo3", "Galvo4", "Digital", "Free", "Loop", "SMoveTime", "Image1X", "Image1Y", "Image2X", "Image2Y"}, dbl}
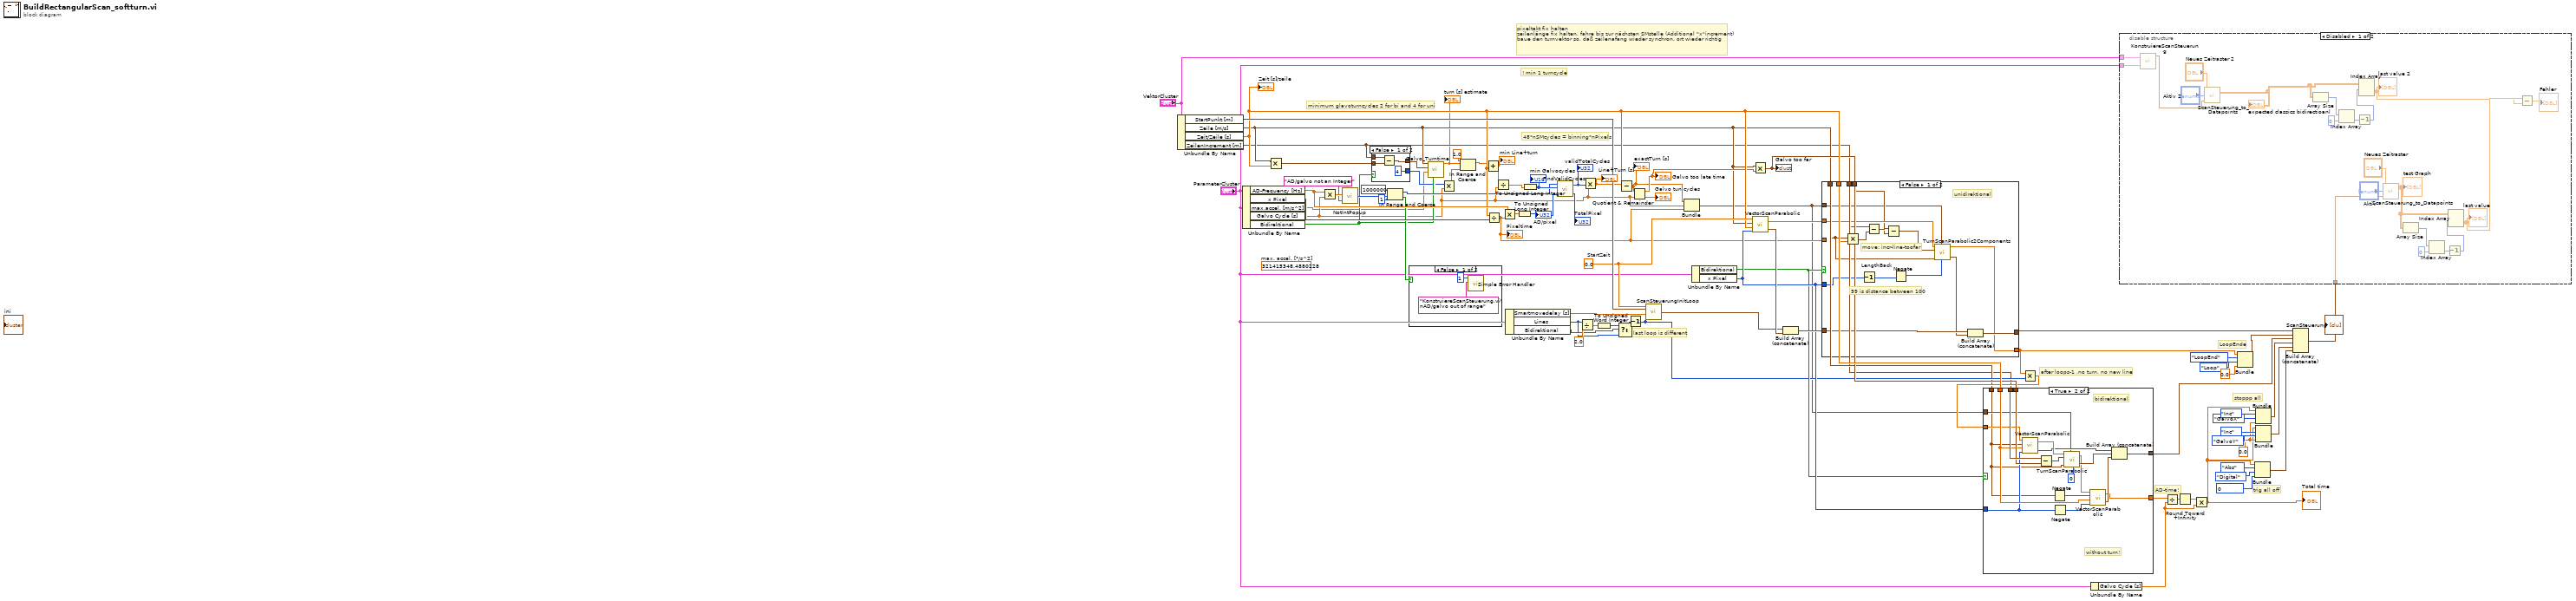
[diagram p0: block diagram]
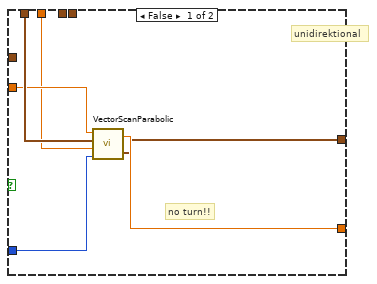
[diagram p4: hidden frame]
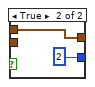
[diagram p5: hidden frame]
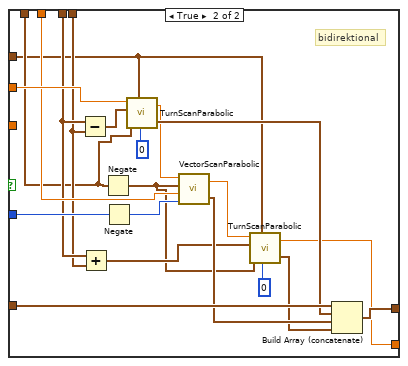
[diagram p6: hidden frame]
diagram:
  (unwired) 321415348.4880228  # max. accel. [°/s^2]
  w32 = 0.0
  w58 = 0.0  # StartZeit
  # "AD-time!"
  # "minimum glavoturncycles 2 for bi and 4 for uni"
  # "after loops-1 ,no turn, no new line"
  # "last loop is different"
  # "! min 1 turncycle"
  # "pixeltakt fix halten\nzeilenlänge fix halten, fahre bis zur nächsten SMstelle (Additional \"x\"increment)\nbaue den turnvektor so, daß zeilenafang wieder synchron, ort wieder richtig"
  # "48*nSMcycles = binning*nPixels"
  # "trig all off"
  # "stoppp all"
  # "LoopEnde"
  n1 = Unbundle By Name("VektorCluster") -> ("StartPunkt [m]"=w59:cluster{"x":dbl, "y":dbl}, "Zeile [m/s]"=w29:cluster{"x":dbl, "y":dbl}, "Zeit/Zeile [s]"=w52:dbl, "ZeilenIncrement [m]"=w28:cluster{"x":dbl, "y":dbl})
  "Zeit [s]/zeile" <- w52
  n2 = Unbundle By Name("ParameterCluster") -> ("AD-Frequency [Hz]"=w60:dbl, "x Pixel"=w67:i32, "max.accel. [m/s^2]"=w8:dbl, "Galvo Cycle [s]"=w18:dbl, "Bidirektional"=w30:bool)
  n3 = Multiply(x=w29, y=w52) -> (x*y=w26:cluster{"x":dbl, "y":dbl})
  n4 = Multiply(x=w60, y=w18) -> (x*y=w43:dbl)
  n5 = call "NotIntPopup.vi"("Err message"="AD/galvo not an Integer", "INT?"=w43) -> ("32bit integer"=w41:i32)  [unwired: 1 in]
  n6 = case shown="False" w30 {
    tunnel: w28 -> [w83 w85]
    tunnel: [w81 w85] -> w27
    tunnel: w26 -> [w82 _]
    tunnel: [4 2] -> w24
    frame False {
      n7 = Subtract(x=w83, y=w82) -> (x-y=w81:cluster{"x":dbl, "y":dbl})
    }
    frame True {
    }
  }
  n8 = In Range and Coerce(upper limit=1000000, x=w41, lower limit=1) -> (coerced(x)=w40:i32, In Range?=w37:bool)
  n9 = case shown="False" w37 {
    frame False {
      n10 = call <vilib>:"Simple Error Handler.vi"("error code (no error:0)"=1, "error source (\" \")"="KonstruiereScanSteuerung.vi\nAD/galvo out of range" ("Err message")) -> ()  [unwired: 2 in, 6 out]
    }
    frame True {
    }
  }
  n11 = call "Galvo_Turntime.vi"("bidirectional"=w30, "Maximal acceleration [m/s^2]"=w8, "delta x [m]"=w27, "start-speed [m/s]"=w29) -> ("duration [s]"=w7:dbl)  [unwired: 1 in, 6 out]
  "turn [s] estimate" <- w7
  n12 = Multiply(x=w24, y=w18) -> (x*y=w22:dbl)
  n13 = In Range and Coerce(upper limit=1.0, x=w7, lower limit=w22) -> (coerced(x)=w23:dbl)  [unwired: 1 out]
  n14 = Add(x=w23, y=w52) -> (x+y=w55:dbl)
  "min Line+turn" <- w55
  n15 = Divide(x=w52, y=w67) -> (x/y=w17:dbl)
  "Pixeltime" <- w17
  n16 = Divide(x=w55, y=w18) -> (x/y=w20:dbl)
  n17 = Multiply(x=w60, y=w17) -> (x*y=w61:dbl)
  n18 = Unbundle By Name("ParameterCluster") -> ("Smartmovedelay [s]"=w57:dbl, "Lines"=w10:i32, "Bidirektional"=w11:bool)
  n19 = To Unsigned Long Integer(number=w61) -> (unsigned 32bit integer=w62:u32)
  "AD/pixel" <- w62
  n20 = To Unsigned Long Integer(number=w20) -> (unsigned 32bit integer=w64:u32)
  "min Galvocycles" <- w64
  n21 = call "FindValidCycles.vi"("C (Fix)"=w62, "B (+x)"=w64, "A (Fix)"=w40) -> ("D"=→"TotalPixel":u32, "B Out"=w54:u32)
  "validTotalCycles" <- w54
  n22 = Divide(x=w10, y=2.0) -> (x/y=w13:dbl)
  n23 = Multiply(x=w18, y=w54) -> (x*y=w53:dbl)
  "Line+Turn [s]" <- w53
  n24 = To Unsigned Word Integer(number=w13) -> (unsigned 16bit integer=w12:u16)
  n25 = Select(t=w12, s=w11, f=w10) -> (s? t:f=w9:i32)
  n26 = Subtract(x=w53, y=w52) -> (x-y=w19:dbl)
  "exactTurn [s]" <- w19
  n27 = Decrement(x=w9) -> (x-1=w44:i32)
  n28 = Quotient & Remainder(x=w19, y=w18) -> (x-y*floor(x/y)=w50:dbl, floor(x/y)=→"Galvo tun cycles":dbl)
  "Galvo too late time" <- w50
  n29 = call "ScanSteuerungInitLoop.vi"("Loops"=w44, "Smartmovedelay [s]"=w57, "StartPunkt [m]"=w59, "StartZeit"=w58) -> ("ScanSteuerung"=w56:T8)
  n30 = Bundle(w19, "Galvo Cycle [s]"=w18, w17) -> (w16:cluster{dbl, "Galvo Cycle [s]":dbl, dbl})  [unwired: 1 out]
  n31 = Unbundle By Name("ParameterCluster") -> ("Bidirektional"=w48:bool, "x Pixel"=w49:i32)
  n32 = call "VectorScanParabolic.vi"("Pixel"=w49, "Zeit/zeile [s]"=w52, "Zeile [m/s]"=w29, "StartZeit"=w58) -> ("ScanSteuerung"=w66:T4, "EndZeit"=w65:dbl)
  n33 = Multiply(x=w29, y=w50) -> (x*y=w51:cluster{"x":dbl, "y":dbl})
  "Galvo too far" <- w51
  n34 = Build Array (concatenate)(w56, w66) -> (w79:T8)
  n35 = case shown="False" w48 {
    tunnel: w79 -> [w103 w124]
    tunnel: [w102 w123] -> w78
    tunnel: w29 -> [w90 w106]
    tunnel: w49 -> [w93 w122]
    tunnel: w28 -> [w101 w108]
    tunnel: w52 -> [w96 w111]
    tunnel: [w100 w116] -> w71
    tunnel: w65 -> [w97 w115]
    tunnel: w51 -> [w94 w107]
    tunnel: w17 -> [_ _]
    tunnel: w16 -> [w88 w104]
    frame False {
      # "99 is distance between 100"
      # "unidirektional"
      # "move: incr-line-toofar"
      n36 = Multiply(x=w90, y=w96) -> (x*y=w95:cluster{"x":dbl, "y":dbl})
      n37 = Decrement "LengthBack"(x=w93) -> (x-1=w92:i32)
      n38 = Subtract(x=w101, y=w95) -> (x-y=w99:cluster{"x":dbl, "y":dbl})
      n39 = Subtract(x=w99, y=w94) -> (x-y=w91:cluster{"x":dbl, "y":dbl})
      n40 = Negate(x=w92) -> (-x=w89:i32)
      n41 = call "TurnScanParabolic2Components.vi"("Start [s] AD raster"=w97, "TurnParameters"=w88, "deltaPosition [m]"=w91, "xPixel"=w89, "speed [m/s]"=w90) -> ("Ende [s] AD+g raster"=w100:dbl, "ScanSteuerung"=w98:T4)  [unwired: 2 in]
      n42 = Build Array (concatenate)(w103, w98) -> (w102:T8)
    }
    frame True {
      # "bidirektional"
      n43 = Subtract(x=w108, y=w107) -> (x-y=w110:cluster{"x":dbl, "y":dbl})
      n44 = Add(x=w108, y=w107) -> (x+y=w109:cluster{"x":dbl, "y":dbl})
      n45 = Negate(x=w106) -> (-x=w105:cluster{"x":dbl, "y":dbl})
      n46 = Negate(x=w122) -> (-x=w112:i32)
      n47 = call "TurnScanParabolic.vi"("xPixel"=0 ("Galvo"), "TurnParameters"=w104, "Zeile [m/s]"=w106, "corrZeilenIncrement [m]"=w110, "Start [s] AD raster"=w115) -> ("ScanSteuerung"=w120:T4, "Ende [s] AD+g raster"=w119:dbl)  [unwired: 1 in]
      n48 = call "VectorScanParabolic.vi"("Pixel"=w112, "Zeit/zeile [s]"=w111, "Zeile [m/s]"=w105, "StartZeit"=w119) -> ("ScanSteuerung"=w121:T4, "EndZeit"=w118:dbl)
      n49 = call "TurnScanParabolic.vi"("xPixel"=0 ("Galvo"), "TurnParameters"=w104, "Zeile [m/s]"=w105, "corrZeilenIncrement [m]"=w109, "Start [s] AD raster"=w118) -> ("ScanSteuerung"=w117:T4, "Ende [s] AD+g raster"=w116:dbl)  [unwired: 1 in]
      n50 = Build Array (concatenate)(w124, w120, w121, w117) -> (w123:T8)
    }
  }
  n51 = Multiply(x=w71, y=w44) -> (x*y=w47:dbl)
  n52 = case shown="True" w48 {
    tunnel: [w127 w148] -> w45
    tunnel: w29 -> [w130 w131]
    tunnel: w49 -> [w126 w134]
    tunnel: w28 -> [_ w140]
    tunnel: w52 -> [w125 w137]
    tunnel: [w128 w138] -> w5
    tunnel: w47 -> [w129 w136]
    tunnel: w51 -> [_ w139]
    tunnel: w16 -> [_ w132]
    frame False {
      # "no turn!!"
      # "unidirektional"
      n53 = call "VectorScanParabolic.vi"("Pixel"=w126, "Zeit/zeile [s]"=w125, "Zeile [m/s]"=w130, "StartZeit"=w129) -> ("ScanSteuerung"=w127:T4, "EndZeit"=w128:dbl)
    }
    frame True {
      # "without turn!"
      # "bidirektional"
      n54 = call "VectorScanParabolic.vi"("Pixel"=w134, "Zeit/zeile [s]"=w137, "Zeile [m/s]"=w131, "StartZeit"=w136) -> ("ScanSteuerung"=w133:T4, "EndZeit"=w135:dbl)
      n55 = Subtract(x=w140, y=w139) -> (x-y=w141:cluster{"x":dbl, "y":dbl})
      n56 = Negate(x=w131) -> (-x=w143:cluster{"x":dbl, "y":dbl})
      n57 = Negate(x=w134) -> (-x=w142:i32)
      n58 = call "TurnScanParabolic.vi"("xPixel"=0 ("Galvo"), "TurnParameters"=w132, "Zeile [m/s]"=w131, "corrZeilenIncrement [m]"=w141, "Start [s] AD raster"=w135) -> ("ScanSteuerung"=w146:T4, "Ende [s] AD+g raster"=w145:dbl)  [unwired: 1 in]
      n59 = call "VectorScanParabolic.vi"("Pixel"=w142, "Zeit/zeile [s]"=w137, "Zeile [m/s]"=w143, "StartZeit"=w145) -> ("ScanSteuerung"=w147:T4, "EndZeit"=w138:dbl)
      n60 = Build Array (concatenate)(w133, w146, w147) -> (w148:T4)
    }
  }
  n61 = Unbundle By Name("ParameterCluster") -> ("Galvo Cycle [s]"=w1:dbl)
  n62 = Divide(x=w5, y=w1) -> (x/y=w4:dbl)
  n63 = Round Toward +Infinity(x=w4) -> (ceil(x): smallest int >= x=w3:dbl)
  n64 = Multiply(x=w3, y=w1) -> (x*y=w6:dbl)
  "Total time" <- w6
  n65 = Bundle("Ende [s] AD+g raster"=w71, "Wirkung"=T7."LoopEnd", "Kanal"=T6."Loop", 0.0) -> (w76:T11)  [unwired: 1 out]
  n66 = Bundle(w6, "Wirkung"=T7."Abs", "Kanal"=T6."Digital", u8 0) -> (w68:T12)  [unwired: 1 out]
  n67 = Bundle(w6, "Wirkung"=T7."Inc", "Kanal"=T6."GalvoX", w32) -> (w46:T13)  [unwired: 1 out]
  n68 = Bundle(w6, "Wirkung"=T7."Inc", "Kanal"=T6."GalvoY", w32) -> (w72:T13)  [unwired: 1 out]
  n69 = Build Array (concatenate)(w78, w76, w45, w46, w72, w68) -> (w15:T8)
  "ScanSteuerung" <- w15
  n70 = disable-structure shown="Disabled" {
    disable-tunnel: "VektorCluster" -> [w156 _]
    disable-tunnel: "ParameterCluster" -> [w155 _]
    disable-tunnel: w15 -> [w149 _]
    frame Disabled {
      n71 = call "KonstruiereScanSteuerung.vi"("VektorCluster"=w156, "ParameterCluster"=w155) -> ("ScanSteuerung"=w152:T4)  [unwired: 2 out]
      n72 = call "ScanSteuerung_to_Datapoints.vi"("ScanSteuerung"=w152, "Aktiv"="Aktiv 2", "Neues Zeitraster"="Neues Zeitraster 2") -> ("Waveform Graph"=w151:dbl[][])  [unwired: 1 in, 1 out]
      "expected classics bidirectioanl" <- w151
      n73 = Array Size(array=w151) -> (size(s)=w162:i32[])
      n74 = Index Array(array=w162, index=0) -> (element=w160:i32)
      n75 = Decrement(x=w160) -> (x-1=w150:i32)
      n76 = Index Array(array=w151, index (row)=w150) -> (element=w158:dbl[])  [unwired: 1 in]
      "last value 2" <- w158
      n77 = call "ScanSteuerung_to_Datapoints.vi"("ScanSteuerung"=w149, "Aktiv"="Aktiv", "Neues Zeitraster"="Neues Zeitraster") -> ("Waveform Graph"=w167:dbl[][])  [unwired: 1 in, 1 out]
      "test Graph" <- w167
      n78 = Array Size(array=w167) -> (size(s)=w166:i32[])
      n79 = Index Array(array=w166, index=0) -> (element=w164:i32)
      n80 = Decrement(x=w164) -> (x-1=w163:i32)
      n81 = Index Array(array=w167, index (row)=w163) -> (element=w159:dbl[])  [unwired: 1 in]
      "last value" <- w159
      n82 = Subtract(x=w159, y=w158) -> (x-y=→"Fehler":dbl[])
    }
    frame Enabled {
    }
  }
